vi "4.0.0_Self Test.vi"(7 "Data in":T1, 8 "error in (no error)":errorcluster, 9 "AllControls In":T2, 10 "?":T3, 11 "Message Queue out":T4) -> (0 "error out":errorcluster, 1 "Flow":string, 2 "Data":T3, 3 "Message Queue Out":T4, 5 "Data out":T1)   [LabVIEW 2017]
uses:
  Depends/AMC/subVIs/TypeDefs/amc_Message Queue.ctl
  Depends/AMC/subVIs/TypeDefs/amc_Message.ctl
  Depends/Tools/Keyed Array/Tools_KeyedArray KeyedArray.ctl
  Ctrls/Data.ctl
  Ctrls/AllControls.ctl
  Ctrls/CSV_Data.ctl
  DIPC 692 Daemon API/typdef/destination.ctl
  DIPC 692 Daemon API/typdef/device_mode.ctl
  Ctrls/PathChoose.ctl
  DIPC 692 Daemon API/typdef/read_nvm_section.ctl
  DIPC 692 Daemon API/typdef/get_parameter.ctl
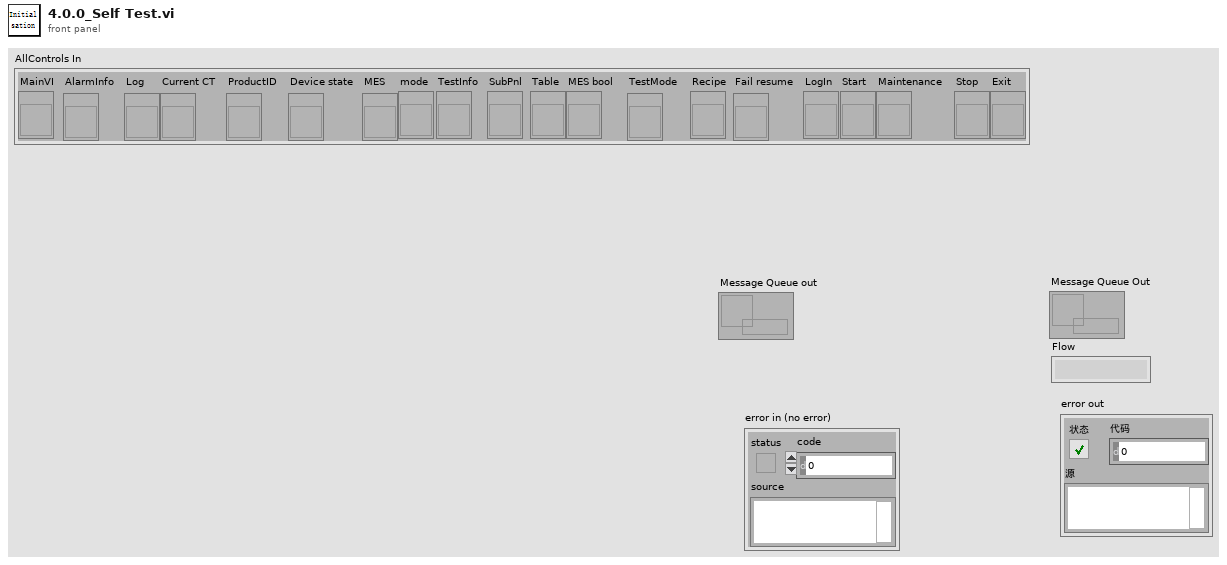
[diagram p1: front panel]
types:
  T1 = typedef "CSV_Data.ctl" = cluster{"Initialisation":cluster{"LMT - Connect UUT (con COM)":string, "LMT - Software Version (rrel)":string, "LMT - Write SKU file (wskuc)":string, "LMT - SKU file name":string, "Connect UUT DDM":string, "Read DDM EOL Timestamp - Mode":string, "Read DDM EOL Timestamp - Timestamp":string, "Read DDM EOL Timestamp - Rig ID":string, "Read DDM EOL Timestamp - Passmark ID":string, "Read DDM EOL Timestamp - Passmark Rev":string, "Software Version before flashing":string, "Read Hardware Serial":string, "UUT DDM SN":string, "Compare DDM SN with MES SN":string, "Backup PCBA Calibration EEPROM Response - CAL":string, "Flash Firmware Version":string, "Check SW Version":string, "Read DDM SW Version after flashing":string, "Set SKU Config":string, "Ready Status":string, "Set Device Mode to EOL":string, "DDM Parameter - Voltage":string, "DDM Parameter - Current":string, "DDM Parameter - Power":string, "DDM Parameter - Speed":string, "DDM Parameter - Pressure":string, "Tester Parameter - Voltage":string, "Tester Parameter - Current":string, "Tester Parameter - Power":string, "Tester Parameter - Ambient Pressure":string, "Tester Parameter - Ambient Temperature":string, "Calculated Parameter - DDM Pressure Corrected":string, "Calculated Parameter - DDM Real Power":string, "Calculated Parameter - Delta V":string}, "BEMF_Calibration":cluster{"Calibration Result - eol_cold_bemf_temp":string, "DDM Ambient Temp":string, "Restriction Plate Diameter":string, "Calibration Result - eol_bemf_mp_cold_coef_a":string, "Calibration Result - eol_bemf_mp_cold_coef_b":string, "Calibration Result - eol_bemf_mp_cold_coef_c":string, "Calibration Result - eol_bemf_lsi_cold_ref_coeffs":string, "Get - Calibration Result - eol_bemf_lsi_speed":string, "Get - Calibration Result - eol_bemf_lsi_integral_0":string, "Calibration Result - eol_bemf_lsi_integral_1":string, "Get - Calibration Result - eol_bemf_lsi_integral_2":string, "Get - Calibration Result - eol_cold_bemf":string, "Get - Calibration Result - eol_cold_bemf_fisf":string, "Finalise Calibration":string, "Compare -Calibration Result - eol_cold_bemf":string, "Compare -Calibration Result - eol_cold_bemf_fisf":string}, "ECO":cluster{"Reset Power Tune":string, "Reset BEMF FISF Calibration":string, "Restriction Plate Diameter":string, "ECO - Stabilisation Time":string, "ECO - DDM Parameter - Voltage":string, "ECO - DDM Parameter - Current":string, "ECO - DDM Parameter - Power":string, "ECO - DDM Parameter - Measured Power":string, "ECO - DDM Parameter - Speed":string, "ECO - DDM Parameter - Pressure":string, "ECO - Tester Parameter - Voltage":string, "ECO - Tester Parameter - Current":string, "ECO - Tester Parameter - Power":string, "ECO - Tester Parameter - Ambient Pressure":string, "ECO - Tester Parameter - Ambient Temperature":string, "ECO - Tester Parameter - Ambient Humidity":string, "ECO - Calculated Parameter - DDM Pressure Corrected":string, "ECO - Calculated Parameter - DDM Real Power":string, "ECO - Calculated Parameter - Delta V":string, "ECO - Calculated Parameter - Flowrate":string, "ECO - Calculated Parameter - Airwatt":string, "ECO - Formula":string, "PT ECO - Power Tune Mode Status":string}, "BOOST":cluster{"Restriction Plate Diameter":string, "BOOST - Stabilisation Time":string, "BOOST - DDM Parameter - Voltage":string, "BOOST - DDM Parameter - Current":string, "BOOST - DDM Parameter - Power":string, "BOOST - DDM Parameter - Measured Power":string, "BOOST - DDM Parameter - Speed":string, "BOOST - DDM Parameter - Pressure":string, "BOOST - Tester Parameter - Voltage":string, "BOOST - Tester Parameter - Current":string, "BOOST - Tester Parameter - Power":string, "BOOST - Tester Parameter - Ambient Pressure":string, "BOOST - Tester Parameter - Ambient Temperature":string, "BOOST - Tester Parameter - Ambient Humidity":string, "BOOST - Calculated Parameter - DDM Pressure Corrected":string, "BOOST - Calculated Parameter - DDM Real Power":string, "BOOST - Calculated Parameter - Delta V":string, "BOOST - Calculated Parameter - Flowrate":string, "BOOST - Calculated Parameter - Airwatt":string, "BOOST - Get AM Presence":string, "Air Muscle Turn Off Status":string, "BOOST - Air Muscle Calculated Parameter - Airwatt B":string, "BOOST - Air Muscle Calculate Airwatt Delta":string, "PT BOOST - Power Tune Mode Status":string, "Finalise Calibration":string, "ECO - Get AW Calibration value":string, "BOOST - Get AW Calibration value":string}, "MAX":cluster{"Restriction Plate Diameter":string, "MAX - Stabilisation Time":string, "Get Average Delta Tmag (LSIdelta_FISFdelta_LSItmag_FISFtmag_IIRtmag)":string, "Get Average Delta Tmag FISF":string, "MAX - DDM Parameter - Voltage":string, "MAX - DDM Parameter - Current":string, "MAX - DDM Parameter - Power":string, "MAX - DDM Parameter - Measured Power":string, "MAX - DDM Parameter - Speed":string, "MAX - DDM Parameter - Pressure":string, "MAX - Tester Parameter - Voltage":string, "MAX - Tester Parameter - Current":string, "MAX - Tester Parameter - Power":string, "MAX - Tester Parameter - Ambient Pressure":string, "MAX - Tester Parameter - Ambient Temperature":string, "MAX - Tester Parameter - Ambient Humidity":string, "MAX - Calculated Parameter - DDM Pressure Corrected":string, "MAX - Calculated Parameter - DDM Real Power":string, "MAX - Calculated Parameter - Delta V":string, "MAX - Calculated Parameter - Flowrate":string, "MAX - Calculated Parameter - Airwatt":string, "MAX_FISF_Check_Average_Delta_Tmag":string, "MAX - FISF - BEMF Finetune Result":string, "MAX tune - Delta P1":string, "MAX tune - Calculated Parameter - Airwatt":string, "Calculate Delta Airwatts - MAX finetune - Delta P2":string, "MAX finetune - DDM Parameter - Voltage":string, "MAX finetune - DDM Parameter - Current":string, "MAX finetune - DDM Parameter - Power":string, "MAX finetune - DDM Parameter - Measured Power":string, "MAX finetune - DDM Parameter - Speed":string, "MAX finetune - DDM Parameter - Pressure":string, "MAX finetune - Tester Parameter - Voltage":string, "MAX finetune - Tester Parameter - Current":string, "MAX finetune - Tester Parameter - Power":string, "MAX finetune - Tester Parameter - Ambient Pressure":string, "MAX finetune - Tester Parameter - Ambient Temperature":string, "MAX finetune - Tester Parameter - Ambient Humidity":string, "MAX finetune - Calculated Parameter - DDM Pressure Corrected":string, "MAX finetune - Calculated Parameter - DDM Real Power":string, "MAX finetune - Calculated Parameter - Delta V":string, "MAX finetune - Calculated Parameter - Flowrate":string, "MAX finetune - Calculated Parameter - Airwatt":string, "Check Derate Result":string, "Delta Tmag FISF":string, "Get Hot BEMF Result":string, "Calculate delta Pressure":string, "Finalise Calibration":string, "Calculate & Check Delta BEMF":string, "Delta P Airwatts Value":string}, "LL":cluster{"DDM Ambient Temp":string, "Restriction Plate Diameter":string, "LL - DDM Parameter - Voltage":string, "LL - DDM Parameter - Current":string, "LL - DDM Parameter - Power":string, "LL - DDM Parameter - Measured Power":string, "LL - DDM Parameter - Speed":string, "LL - DDM Parameter - Pressure":string, "LL - Tester Parameter - Voltage":string, "LL - Tester Parameter - Current":string, "LL - Tester Parameter - Power":string, "LL - DDM Real Power":string, "LL - Calibrate Task Detect LL":string}, "HL":cluster{"HL - DDM Parameter - Voltage":string, "HL - DDM Parameter - Current":string, "HL - DDM Parameter - Power":string, "HL - DDM Parameter - Measured Power":string, "HL - DDM Parameter - Speed":string, "HL - DDM Parameter - Pressure":string, "HL - Tester Parameter - Voltage":string, "HL - Tester Parameter - Current":string, "HL - Tester Parameter - Power":string, "HL - DDM Real Power":string, "HL - Calibrate Task Detect HL":string}, "LH":cluster{"Restriction Plate Diameter":string, "LH - DDM Parameter - Voltage":string, "LH - DDM Parameter - Current":string, "LH - DDM Parameter - Power":string, "LH - DDM Parameter - Measured Power":string, "LH - DDM Parameter - Speed":string, "LH - DDM Parameter - Pressure":string, "LH - Tester Parameter - Voltage":string, "LH - Tester Parameter - Current":string, "LH - Tester Parameter - Power":string, "LH - DDM Real Power":string, "LH - Calibrate Task Detect LH":string}, "HH":cluster{"HH - DDM Parameter - Voltage":string, "HH - DDM Parameter - Current":string, "HH - DDM Parameter - Power":string, "HH - DDM Parameter - Measured Power":string, "HH - DDM Parameter - Speed":string, "HH - DDM Parameter - Pressure":string, "HH - Tester Parameter - Voltage":string, "HH - Tester Parameter - Current":string, "HH - Tester Parameter - Power":string, "HH - DDM Real Power":string, "HH - Calibrate Task Detect HH":string}, "Inlet Blockage Calibration":cluster{"Inlet Blockage Calibration - DDM Parameter - Voltage":string, "Inlet Blockage Calibration - DDM Parameter - Current":string, "Inlet Blockage Calibration - DDM Parameter - Power":string, "Inlet Blockage Calibration - DDM Parameter - Measured Power":string, "Inlet Blockage Calibration - DDM Parameter - Speed":string, "Inlet Blockage Calibration - DDM Parameter - Pressure":string, "Inlet Blockage Calibration - Tester Parameter - Voltage":string, "Inlet Blockage Calibration - Tester Parameter - Current":string, "Inlet Blockage Calibration - Tester Parameter - Power":string, "Inlet Blockage Calibration - DDM Real Power":string, "Calibration Inlet Blockage_E":string, "Finalise Calibration":string, "Get Task Detect LL":string, "Get Task Detect HL":string, "Get Task Detect LH":string, "Get Task Detect HH":string, "Calibration Inlet Blockage":string, "Calibration eol cold bemf temp":string}, "GOOD":cluster{"GOOD UNIT - Clear EEPROM Error Log":string, "GOOD UNIT - Write Product Timestamp - Mode":string, "GOOD UNIT - Write Product Timestamp - Timestamp":string, "GOOD UNIT - Write Product Timestamp - Rig ID":string, "GOOD UNIT - Write Product Timestamp - Passmark ID":string, "GOOD UNIT - Write Product Timestamp - Passmark Rev":string, "GOOD UNIT - Set Device Mode to PROD":string, "GOOD UNIT - Backup PCBA Calibration EEPROM Response":string, "GOOD UNIT - Check Security Bit":string, "GOOD UNIT - Set Calibration Lock":string, "GOOD UNIT - Get_Calibration_Lock":string, "GOOD UNIT - Disconnect UUT":string}, "NG":cluster{"NG UNIT - Read NVM Error":string, "NG UNIT - Set Device Mode to FCT":string, "NG UNIT - Backup PCBA Calibration EEPROM Response - CAL":string, "NG UNIT - Backup PCBA Calibration EEPROM Response - ERROR":string, "NG UNIT - Backup PCBA Calibration EEPROM Response - USAGE":string, "NG UNIT - Disconnect UUT":string}, "SN":string, "Table":string[][], "Count":cluster{"Total":i32, "OK":i32, "NG":i32, "Yield":dbl}, "Start Time":timestamp, "daemon reference":refnum<k5>, "CT":dbl, "Config":string[][], "OK/NG":bool, "Station ID":string, "MES DDM SN":string, "MES PCBA SN":string, "Retest":string, "Lux":string, "Initialisation_Status":cluster{"LMT - Connect UUT (con COM)":string, "LMT - Software Version (rrel)":string, "LMT - Write SKU file (wskuc)":string, "LMT - SKU file name":string, "Connect UUT DDM":string, "Read DDM EOL Timestamp - Mode":string, "Read DDM EOL Timestamp - Timestamp":string, "Read DDM EOL Timestamp - Rig ID":string, "Read DDM EOL Timestamp - Passmark ID":string, "Read DDM EOL Timestamp - Passmark Rev":string, "Software Version before flashing":string, "Read Hardware Serial":string, "UUT DDM SN":string, "Compare DDM SN with MES SN":string, "Backup PCBA Calibration EEPROM Response - CAL":string, "Flash Firmware Version":string, "Check SW Version":string, "Read DDM SW Version after flashing":string, "Set SKU Config":string, "Ready Status":string, "Set Device Mode to EOL":string, "DDM Parameter - Voltage":string, "DDM Parameter - Current":string, "DDM Parameter - Power":string, "DDM Parameter - Speed":string, "DDM Parameter - Pressure":string, "Tester Parameter - Voltage":string, "Tester Parameter - Current":string, "Tester Parameter - Power":string, "Tester Parameter - Ambient Pressure":string, "Tester Parameter - Ambient Temperature":string, "Calculated Parameter - DDM Pressure Corrected":string, "Calculated Parameter - DDM Real Power":string, "Calculated Parameter - Delta V":string}, "BEMF_Calibration_Status":cluster{"Calibration Result - eol_cold_bemf_temp":string, "DDM Ambient Temp":string, "Restriction Plate Diameter":string, "Calibration Result - eol_bemf_mp_cold_coef_a":string, "Calibration Result - eol_bemf_mp_cold_coef_b":string, "Calibration Result - eol_bemf_mp_cold_coef_c":string, "Calibration Result - eol_bemf_lsi_cold_ref_coeffs":string, "Get - Calibration Result - eol_bemf_lsi_speed":string, "Get - Calibration Result - eol_bemf_lsi_integral_0":string, "Calibration Result - eol_bemf_lsi_integral_1":string, "Get - Calibration Result - eol_bemf_lsi_integral_2":string, "Get - Calibration Result - eol_cold_bemf":string, "Get - Calibration Result - eol_cold_bemf_fisf":string, "Finalise Calibration":string, "Compare -Calibration Result - eol_cold_bemf":string, "Compare -Calibration Result - eol_cold_bemf_fisf":string}, "ECO_Status":cluster{"Reset Power Tune":string, "Reset BEMF FISF Calibration":string, "Restriction Plate Diameter":string, "ECO - Stabilisation Time":string, "ECO - DDM Parameter - Voltage":string, "ECO - DDM Parameter - Current":string, "ECO - DDM Parameter - Power":string, "ECO - DDM Parameter - Measured Power":string, "ECO - DDM Parameter - Speed":string, "ECO - DDM Parameter - Pressure":string, "ECO - Tester Parameter - Voltage":string, "ECO - Tester Parameter - Current":string, "ECO - Tester Parameter - Power":string, "ECO - Tester Parameter - Ambient Pressure":string, "ECO - Tester Parameter - Ambient Temperature":string, "ECO - Tester Parameter - Ambient Humidity":string, "ECO - Calculated Parameter - DDM Pressure Corrected":string, "ECO - Calculated Parameter - DDM Real Power":string, "ECO - Calculated Parameter - Delta V":string, "ECO - Calculated Parameter - Flowrate":string, "ECO - Calculated Parameter - Airwatt":string, "ECO - Formula":string, "PT ECO - Power Tune Mode Status":string}, "BOOST_Status":cluster{"Restriction Plate Diameter":string, "BOOST - Stabilisation Time":string, "BOOST - DDM Parameter - Voltage":string, "BOOST - DDM Parameter - Current":string, "BOOST - DDM Parameter - Power":string, "BOOST - DDM Parameter - Measured Power":string, "BOOST - DDM Parameter - Speed":string, "BOOST - DDM Parameter - Pressure":string, "BOOST - Tester Parameter - Voltage":string, "BOOST - Tester Parameter - Current":string, "BOOST - Tester Parameter - Power":string, "BOOST - Tester Parameter - Ambient Pressure":string, "BOOST - Tester Parameter - Ambient Temperature":string, "BOOST - Tester Parameter - Ambient Humidity":string, "BOOST - Calculated Parameter - DDM Pressure Corrected":string, "BOOST - Calculated Parameter - DDM Real Power":string, "BOOST - Calculated Parameter - Delta V":string, "BOOST - Calculated Parameter - Flowrate":string, "BOOST - Calculated Parameter - Airwatt":string, "BOOST - Get AM Presence":string, "Air Muscle Turn Off Status":string, "BOOST - Air Muscle Calculated Parameter - Airwatt B":string, "BOOST - Air Muscle Calculate Airwatt Delta":string, "PT BOOST - Power Tune Mode Status":string, "Finalise Calibration":string, "ECO - Get AW Calibration value":string, "BOOST - Get AW Calibration value":string}, "MAX_Status":cluster{"Restriction Plate Diameter":string, "MAX - Stabilisation Time":string, "Get Average Delta Tmag (LSIdelta_FISFdelta_LSItmag_FISFtmag_IIRtmag)":string, "Get Average Delta Tmag FISF":string, "MAX - DDM Parameter - Voltage":string, "MAX - DDM Parameter - Current":string, "MAX - DDM Parameter - Power":string, "MAX - DDM Parameter - Measured Power":string, "MAX - DDM Parameter - Speed":string, "MAX - DDM Parameter - Pressure":string, "MAX - Tester Parameter - Voltage":string, "MAX - Tester Parameter - Current":string, "MAX - Tester Parameter - Power":string, "MAX - Tester Parameter - Ambient Pressure":string, "MAX - Tester Parameter - Ambient Temperature":string, "MAX - Tester Parameter - Ambient Humidity":string, "MAX - Calculated Parameter - DDM Pressure Corrected":string, "MAX - Calculated Parameter - DDM Real Power":string, "MAX - Calculated Parameter - Delta V":string, "MAX - Calculated Parameter - Flowrate":string, "MAX - Calculated Parameter - Airwatt":string, "MAX_FISF_Check_Average_Delta_Tmag":string, "MAX - FISF - BEMF Finetune Result":string, "MAX tune - Delta P1":string, "MAX tune - Calculated Parameter - Airwatt":string, "Calculate Delta Airwatts - MAX finetune - Delta P2":string, "MAX finetune - DDM Parameter - Voltage":string, "MAX finetune - DDM Parameter - Current":string, "MAX finetune - DDM Parameter - Power":string, "MAX finetune - DDM Parameter - Measured Power":string, "MAX finetune - DDM Parameter - Speed":string, "MAX finetune - DDM Parameter - Pressure":string, "MAX finetune - Tester Parameter - Voltage":string, "MAX finetune - Tester Parameter - Current":string, "MAX finetune - Tester Parameter - Power":string, "MAX finetune - Tester Parameter - Ambient Pressure":string, "MAX finetune - Tester Parameter - Ambient Temperature":string, "MAX finetune - Tester Parameter - Ambient Humidity":string, "MAX finetune - Calculated Parameter - DDM Pressure Corrected":string, "MAX finetune - Calculated Parameter - DDM Real Power":string, "MAX finetune - Calculated Parameter - Delta V":string, "MAX finetune - Calculated Parameter - Flowrate":string, "MAX finetune - Calculated Parameter - Airwatt":string, "Check Derate Result":string, "Delta Tmag FISF":string, "Get Hot BEMF Result":string, "Calculate delta Pressure":string, "Finalise Calibration":string, "Calculate & Check Delta BEMF":string, "Delta P Airwatts Value":string}, "LL_Status":cluster{"DDM Ambient Temp":string, "Restriction Plate Diameter":string, "LL - DDM Parameter - Voltage":string, "LL - DDM Parameter - Current":string, "LL - DDM Parameter - Power":string, "LL - DDM Parameter - Measured Power":string, "LL - DDM Parameter - Speed":string, "LL - DDM Parameter - Pressure":string, "LL - Tester Parameter - Voltage":string, "LL - Tester Parameter - Current":string, "LL - Tester Parameter - Power":string, "LL - DDM Real Power":string, "LL - Calibrate Task Detect LL":string}, "HL_Status":cluster{"HL - DDM Parameter - Voltage":string, "HL - DDM Parameter - Current":string, "HL - DDM Parameter - Power":string, "HL - DDM Parameter - Measured Power":string, "HL - DDM Parameter - Speed":string, "HL - DDM Parameter - Pressure":string, "HL - Tester Parameter - Voltage":string, "HL - Tester Parameter - Current":string, "HL - Tester Parameter - Power":string, "HL - DDM Real Power":string, "HL - Calibrate Task Detect HL":string}, "LH_Status":cluster{"Restriction Plate Diameter":string, "LH - DDM Parameter - Voltage":string, "LH - DDM Parameter - Current":string, "LH - DDM Parameter - Power":string, "LH - DDM Parameter - Measured Power":string, "LH - DDM Parameter - Speed":string, "LH - DDM Parameter - Pressure":string, "LH - Tester Parameter - Voltage":string, "LH - Tester Parameter - Current":string, "LH - Tester Parameter - Power":string, "LH - DDM Real Power":string, "LH - Calibrate Task Detect LH":string}, "HH_Status":cluster{"HH - DDM Parameter - Voltage":string, "HH - DDM Parameter - Current":string, "HH - DDM Parameter - Power":string, "HH - DDM Parameter - Measured Power":string, "HH - DDM Parameter - Speed":string, "HH - DDM Parameter - Pressure":string, "HH - Tester Parameter - Voltage":string, "HH - Tester Parameter - Current":string, "HH - Tester Parameter - Power":string, "HH - DDM Real Power":string, "HH - Calibrate Task Detect HH":string}, "Inlet Blockage Calibration_Status":cluster{"Inlet Blockage Calibration - DDM Parameter - Voltage":string, "Inlet Blockage Calibration - DDM Parameter - Current":string, "Inlet Blockage Calibration - DDM Parameter - Power":string, "Inlet Blockage Calibration - DDM Parameter - Measured Power":string, "Inlet Blockage Calibration - DDM Parameter - Speed":string, "Inlet Blockage Calibration - DDM Parameter - Pressure":string, "Inlet Blockage Calibration - Tester Parameter - Voltage":string, "Inlet Blockage Calibration - Tester Parameter - Current":string, "Inlet Blockage Calibration - Tester Parameter - Power":string, "Inlet Blockage Calibration - DDM Real Power":string, "Calibration Inlet Blockage_E":string, "Finalise Calibration":string, "Get Task Detect LL":string, "Get Task Detect HL":string, "Get Task Detect LH":string, "Get Task Detect HH":string, "Calibration Inlet Blockage":string, "Calibration eol cold bemf temp":string}, "GOOD_Status":cluster{"GOOD UNIT - Clear EEPROM Error Log":string, "GOOD UNIT - Write Product Timestamp - Mode":string, "GOOD UNIT - Write Product Timestamp - Timestamp":string, "GOOD UNIT - Write Product Timestamp - Rig ID":string, "GOOD UNIT - Write Product Timestamp - Passmark ID":string, "GOOD UNIT - Write Product Timestamp - Passmark Rev":string, "GOOD UNIT - Set Device Mode to PROD":string, "GOOD UNIT - Backup PCBA Calibration EEPROM Response":string, "GOOD UNIT - Check Security Bit":string, "GOOD UNIT - Set Calibration Lock":string, "GOOD UNIT - Get_Calibration_Lock":string, "GOOD UNIT - Disconnect UUT":string}, "NG_Status":cluster{"NG UNIT - Read NVM Error":string, "NG UNIT - Set Device Mode to FCT":string, "NG UNIT - Backup PCBA Calibration EEPROM Response - CAL":string, "NG UNIT - Backup PCBA Calibration EEPROM Response - ERROR":string, "NG UNIT - Backup PCBA Calibration EEPROM Response - USAGE":string, "NG UNIT - Disconnect UUT":string}, "SKU":string, "Plate_Diameter":string, "Alarm":string}
  T2 = typedef "AllControls.ctl" = cluster{"MainVI":refnum<vi>, "AlarmInfo":refnum<vi>, "Log":refnum<vi>, "Current CT":refnum<vi>, "ProductID":refnum<vi>, "Device state":refnum<vi>, "MES":refnum<vi>, "mode":refnum<vi>, "TestInfo":refnum<vi>, "SubPnl":refnum<vi>, "Table":refnum<vi>, "MES bool":refnum<vi>, "TestMode":refnum<vi>, "Recipe":refnum<vi>, "Fail resume":refnum<vi>, "LogIn":refnum<vi>, "Start":refnum<vi>, "Maintenance":refnum<vi>, "Stop":refnum<vi>, "Exit":refnum<vi>}
  T3 = typedef "Data.ctl" = cluster{"Initialisation":cluster{"DDM_Parameter":dbl[], "DDM_Parameter_status":bool[], "Get_Tester_Parameter":dbl[], "Get_Tester_Parameter_status":bool[], "Cal_Tester_Parameter":dbl[], "Cal_Tester_Parameter_status":bool[], "sw_version_before_status":bool, "sw_version_after_status":bool, "Set_SKU_Config_With_LMT_status":bool, "FCT_timestamp_status":bool, "LMT_Connect_to_UUT_status":bool}, "BEMF_Calibration":cluster{"Read_ambient_temperature":dbl, "Calibration_Vaule":dbl[], "Calibration_Vaule _B":dbl[], "Calibration_Vaule_status":bool[], "Calibration_Vaule_B_status":bool[]}, "ECO":cluster{"DDM_Parameter":dbl[], "DDM_Parameter_status":bool[], "Get_Tester_Parameter":dbl[], "Get_Tester_Parameter_status":bool[], "Cal_Tester_Parameter":dbl[], "Cal_Tester_Parameter_status":bool[], "DDM_Parameter_after_power_tune":dbl[], "Get_Tester_Parameter_after_power_tune":dbl[], "Cal_Tester_Parameter_after_power_tune":dbl[], "Cal_Tester_Parameter_after_power_tune_status":bool[], "Delta_P":dbl}, "BOOST":cluster{"DDM_Parameter":dbl[], "DDM_Parameter_status":bool[], "Get_Tester_Parameter":dbl[], "Get_Tester_Parameter_status":bool[], "Cal_Tester_Parameter":dbl[], "Cal_Tester_Parameter_status":bool[], "DDM_Parameter_after_power_tune":dbl[], "Get_Tester_Parameter_after_power_tune":dbl[], "Cal_Tester_Parameter_after_power_tune":dbl[], "Cal_Tester_Parameter_after_power_tune_status":bool[], "airwatts_am_off":dbl, "AW_Delta_(AM_on_and_off)":dbl, "AW_Delta_(AM_on_and_off)_Status":bool, "Delta_P":dbl}, "MAX":cluster{"Average_Tmag_Data":cluster{"LSI Delta in degC":dbl, "FISF Delta in degc":dbl, "LSI Tmag in degC":dbl, "Fisf Tmag in degC":dbl, "IIR Tmag in degC":dbl}, "DDM_Parameter":dbl[], "DDM_Parameter_status":bool[], "Get_Tester_Parameter":dbl[], "Get_Tester_Parameter_status":bool[], "Cal_Tester_Parameter":dbl[], "BEMF_Finetune":cluster{"eol_bemf_mp_cold_coef_c":dbl, "eol_cold_bemf_fisf_offset":dbl}, "AW_Tune":cluster{"delta_P1":dbl, "delta_P_Setting":dbl}, "DDM_Parameter_after_Airwatts_Tune":dbl[], "Get_Tester_Parameter_after_Airwatts_Tune":dbl[], "Cal_Tester_Parameter_after_Airwatts_Tune":dbl[], "DDM_Parameter_after_Airwatts_Finetune":dbl[], "Get_Tester_Parameter_after_Airwatts_Finetune":dbl[], "Cal_Tester_Parameter_after_Airwatts_Finetune":dbl[], "AW_Finetune":cluster{"delta_P2":dbl, "delta_P_Setting":dbl}, "Delta_Tmag_after_tune":cluster{"LSI Delta in degC":dbl, "FISF Delta in degc":dbl, "LSI Tmag in degC":dbl, "Fisf Tmag in degC":dbl, "IIR Tmag in degC":dbl}, "Hot Bemf in mV":dbl, "DDM_Pressure":dbl, "Delta_Pressure":dbl, " Cold Bemf in mV":dbl, " delta Bemf":dbl, " delta p":dbl, "Delta_Pressure_status":bool, " delta Bemf_status":bool, "LSI Delta in degC_status":bool, "FISF Delta in degc_status":bool, "Max_check_derate_status_status":bool, "Average_All_data":dbl[][], "Average_Tmag_Data_status":bool[], "Average_Tmag_Data_after_tune_status":bool[], "Cal_Tester_Parameter_status":bool[], "Cal_Tester_Parameter_status_after_Airwatts_Tune":bool[], "Cal_Tester_Parameter_status_after_Airwatts_FineTune":bool[]}, "Task_Detect_Calib":cluster{"LL":cluster{"DDM_Parameter":dbl[], "DDM_Parameter_status":bool[], "Get_Tester_Parameter":dbl[], "Get_Tester_Parameter_status":bool[], "Set_task_detect_A":dbl, "Set_task_detect_A_Status":bool}, "HL":cluster{"DDM_Parameter":dbl[], "DDM_Parameter_status":bool[], "Get_Tester_Parameter":dbl[], "Get_Tester_Parameter_status":bool[], "Set_task_detect_B":dbl, "Set_task_detect_B_Status":bool}, "LH":cluster{"DDM_Parameter":dbl[], "DDM_Parameter_status":bool[], "Get_Tester_Parameter":dbl[], "Get_Tester_Parameter_status":bool[], "Set_task_detect_C":dbl, "Set_task_detect_C_Status":bool}, "HH":cluster{"DDM_Parameter":dbl[], "DDM_Parameter_status":bool[], "Get_Tester_Parameter":dbl[], "Get_Tester_Parameter_status":bool[], "Set_task_detect_D":dbl, "Read_and_check_calibration_Status":bool[], "Set_task_detect_D_Status":bool}, "Get_eol_inlet_blockage_E":dbl, "Calib_vaule":cluster{"Get_task_detect_LL":dbl, "Get_task_detect_HL":dbl, "Get_task_detect_LH":dbl, "Get_task_detect_HH":dbl, "eol_inlet_blockage":dbl, "eol_code_bemf_temp":dbl}, "calibrated temp":dbl, "Inlet_Blockage_Calibration":cluster{"DDM_Parameter":dbl[], "DDM_Parameter_status":bool[], "Get_Tester_Parameter":dbl[], "Get_Tester_Parameter_status":bool[]}, "Get_eol_inlet_blockage_E_Status":bool}, "good":cluster{"Write_Product_TS":cluster{"TIMESTAMP":i64, "RIG_ID":i64, "PASSMARK_ID":i64, "PASSMARK_REV":i64}, "Read_Product_TS":cluster{"TIMESTAMP":i64, "RIG_ID":i64, "PASSMARK_ID":i64, "PASSMARK_REV":i64}, "Good_Check_Secuity_Bit_Stauts":bool}}
  T4 = typedef "amc_Message Queue.ctl" = refnum<queue>
  T5 = cluster{"Brush_ADC.bat":string, "Get Release Version.bat":string, "Getting Software  Version.bat":string, "Pump_ADC.bat":string, "Starting  Pump Motor.bat":string, "Starting  Test Mode.bat":string, "Starting Brush Motor 1.bat":string, "Starting Brush Motor 2.bat":string, "Starting Brush Motor 3.bat":string, "Starting LED Test.bat":string, "Stopping  Brush Motor.bat":string, "Stopping  Pump Motor.bat":string, "Stopping  Test Mode.bat":string, "1":string, "2":string, "3":string, "4":string, "5":string, "6":string, "7":string, "8":string, "9":string, "10":string}
  T6 = typedef "destination.ctl" = string
  T7 = typedef "PathChoose.ctl" = enum16{"OperatorLog", "AutoRunLog", "AlmLog", "TestData", "AllTestData", "backup_nvm", "backup_before_flashing"}
  T8 = enum16{"open", "replace", "create", "open or create", "replace or create", "replace or create with confirmation"}
  T9 = typedef "read_nvm_section.ctl" = enum16{"CAL", "ERROR", "USAGE"}
  T10 = typedef "get_parameter.ctl" = string
  T11 = typedef "HD Config.ctl" = cluster{" PC":cluster{"PC Address":u8[], "PC Port":i32}, "FCO":cluster{"COM":refnum<visa-resource-name>, "Baudrate":u32}, "DC Power ":cluster{"COM":refnum<visa-resource-name>, "Baudrate":u32}, "PW3336":cluster{"COM":refnum<visa-resource-name>, "Baudrate":u32}, "Lefoo":cluster{"COM":refnum<visa-resource-name>, "Baudrate":u32}, "Tempt&Hum":cluster{"COM":refnum<visa-resource-name>, "Baudrate":u32}, "DIPC":cluster{"COM":refnum<visa-resource-name>}, "Daemon":cluster{"IP Address":string, "Port":u16, "Retry":u16}, "URAT":cluster{"COM":refnum<visa-resource-name>, "Baudrate":u32}, "Fail_resume_mode":bool, "GRR":bool}
  T12 = typedef "device_mode.ctl" = enum16{"FCT", "EOL", "PROD"}
  T13 = cluster{"TIMESTAMP":i64, "RIG_ID":i64, "PASSMARK_ID":i64, "PASSMARK_REV":i64}
  T14 = cluster{"TIMESTAMP":string, "RIG_ID":string, "PASSMARK_ID":string, "PASSMARK_REV":string}
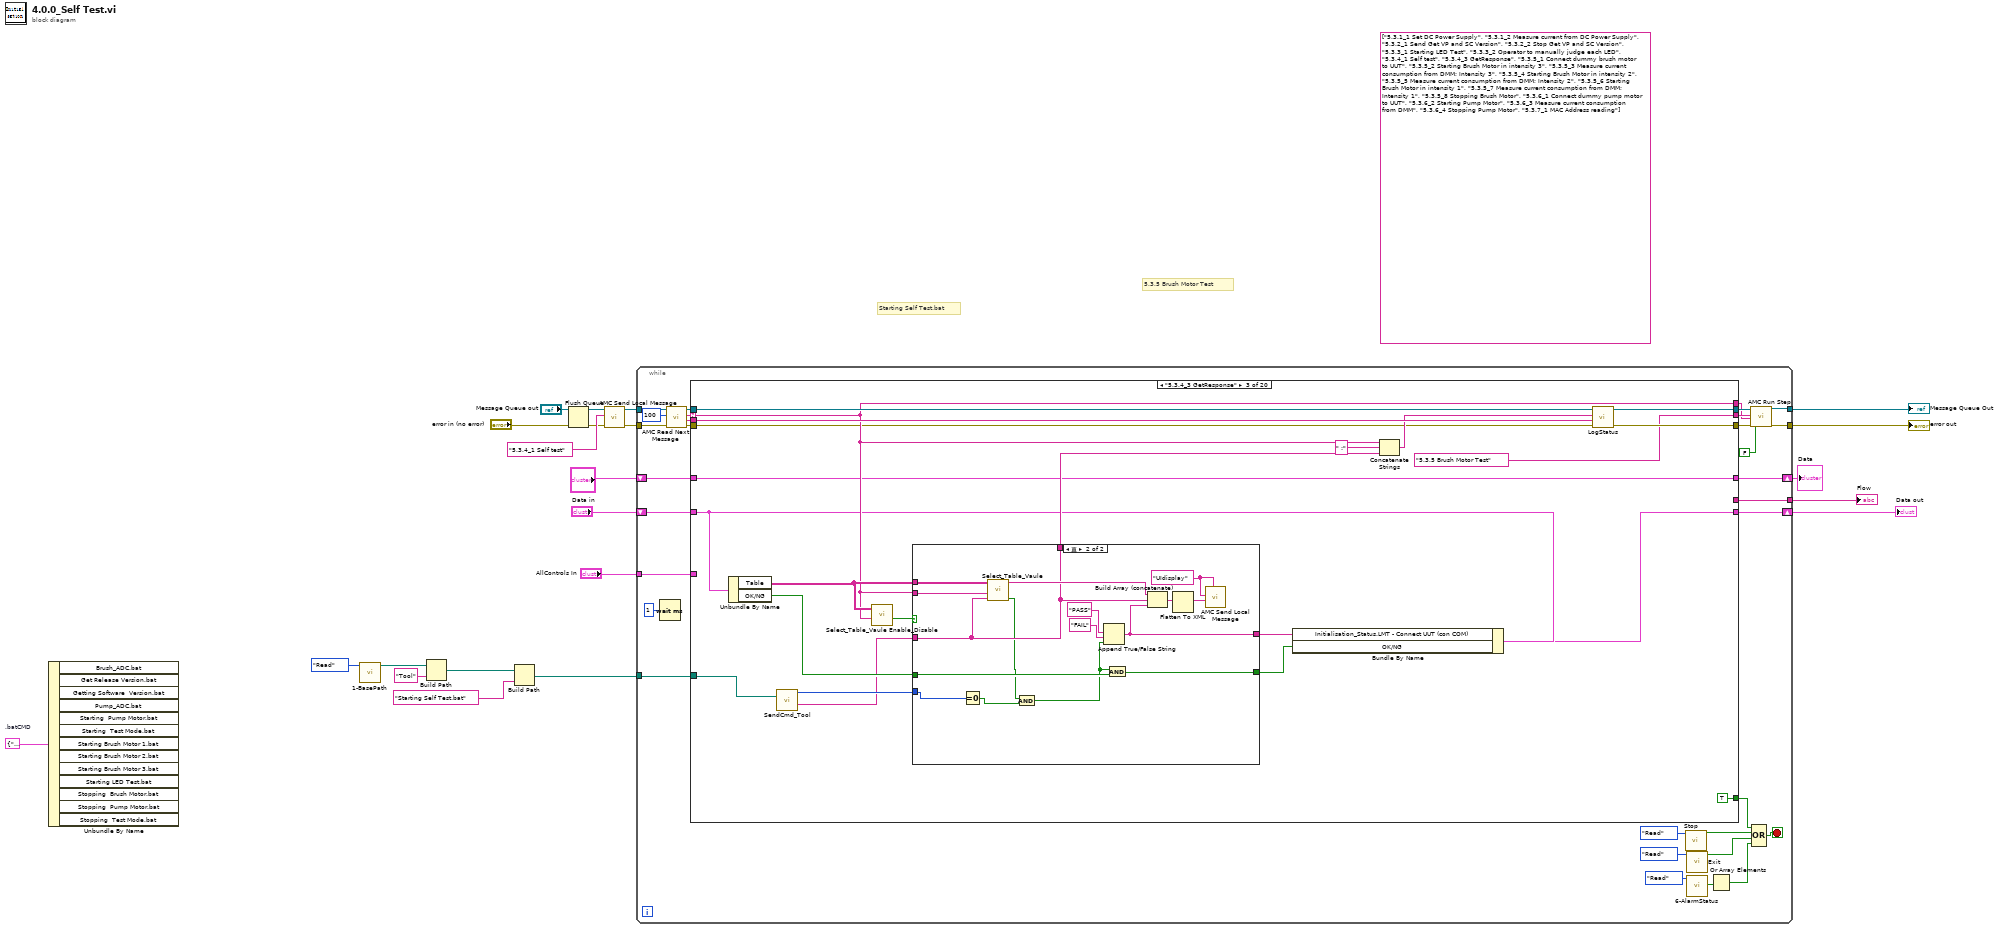
[diagram p0: block diagram]
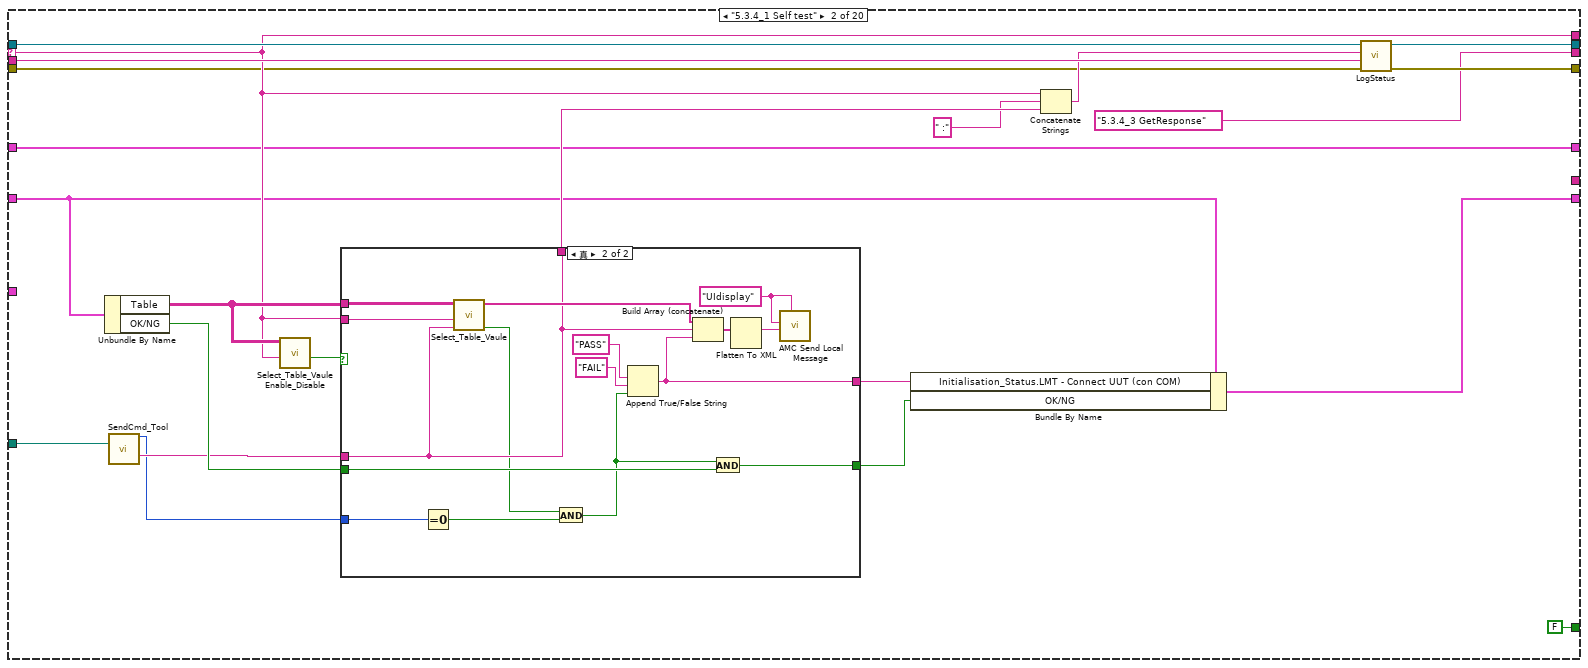
[diagram p3: hidden frame]
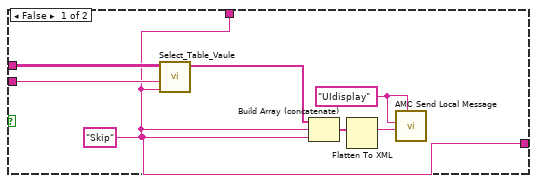
[diagram p4: hidden frame]
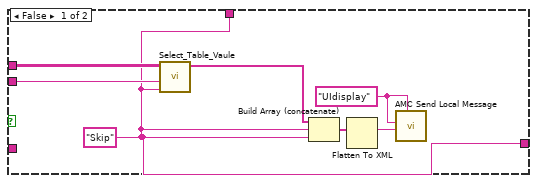
[diagram p5: hidden frame]
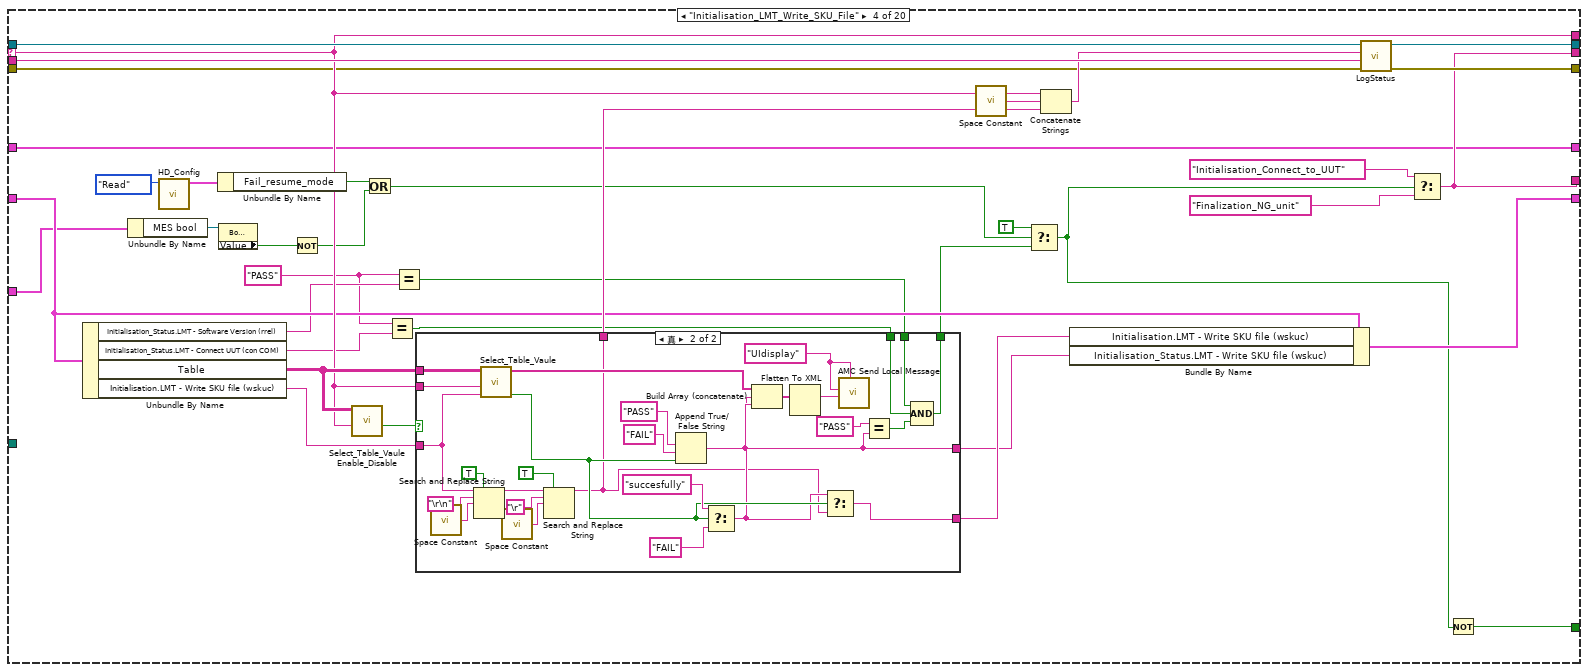
[diagram p6: hidden frame]
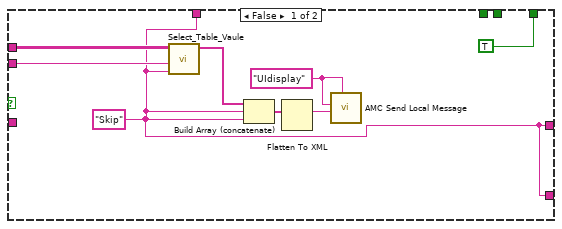
[diagram p7: hidden frame]
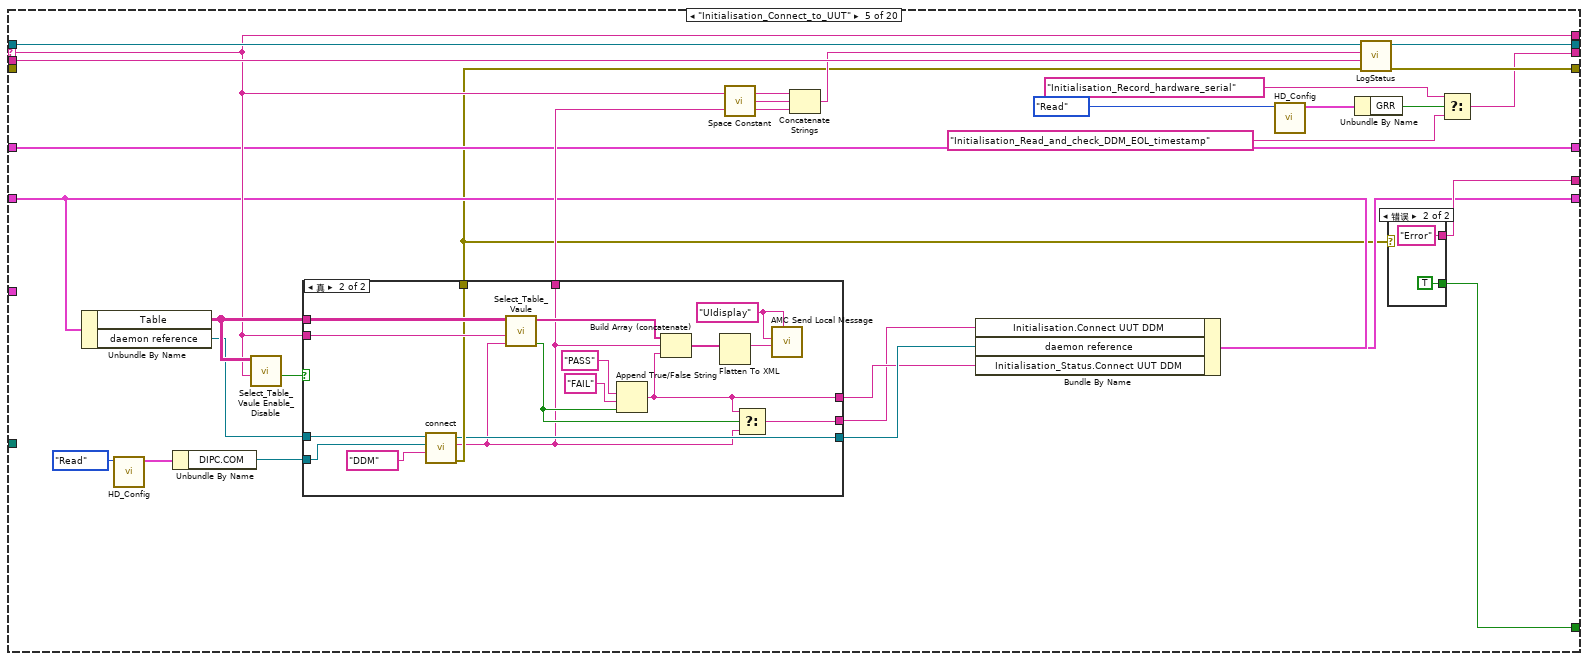
[diagram p8: hidden frame]
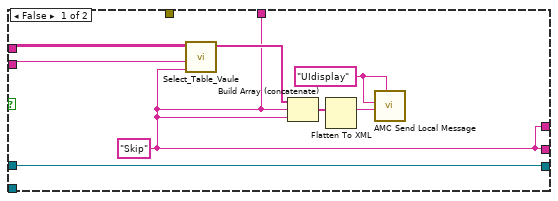
[diagram p10: hidden frame]
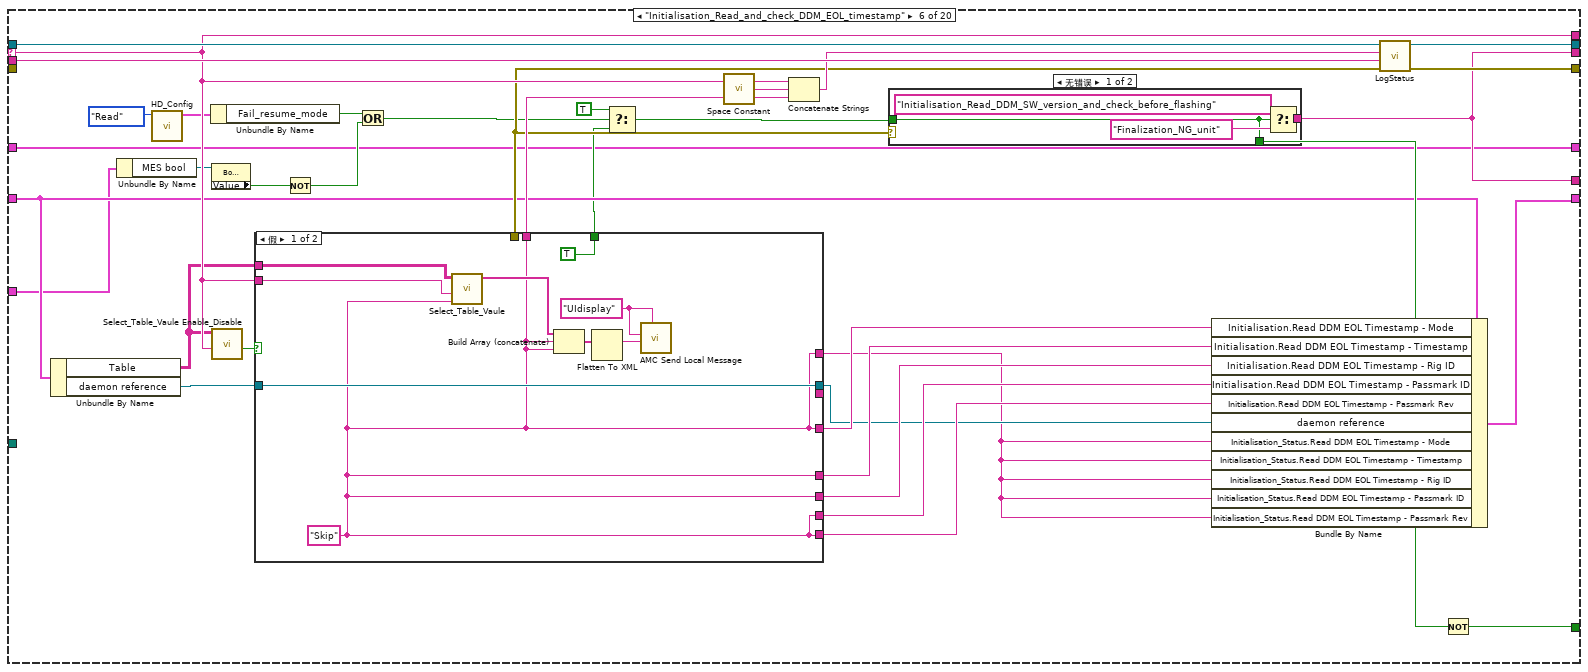
[diagram p11: hidden frame]
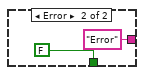
[diagram p12: hidden frame]
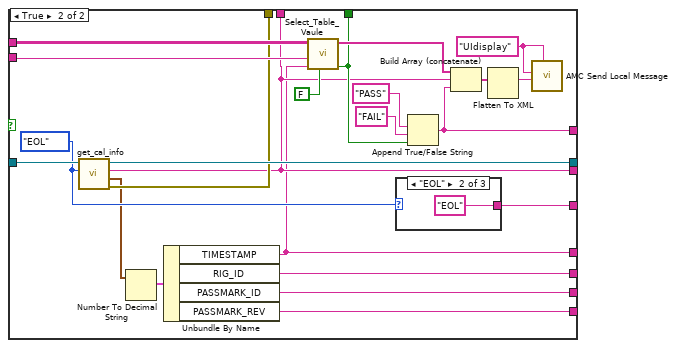
[diagram p13: hidden frame]
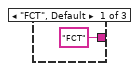
[diagram p14: hidden frame]
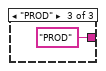
[diagram p15: hidden frame]
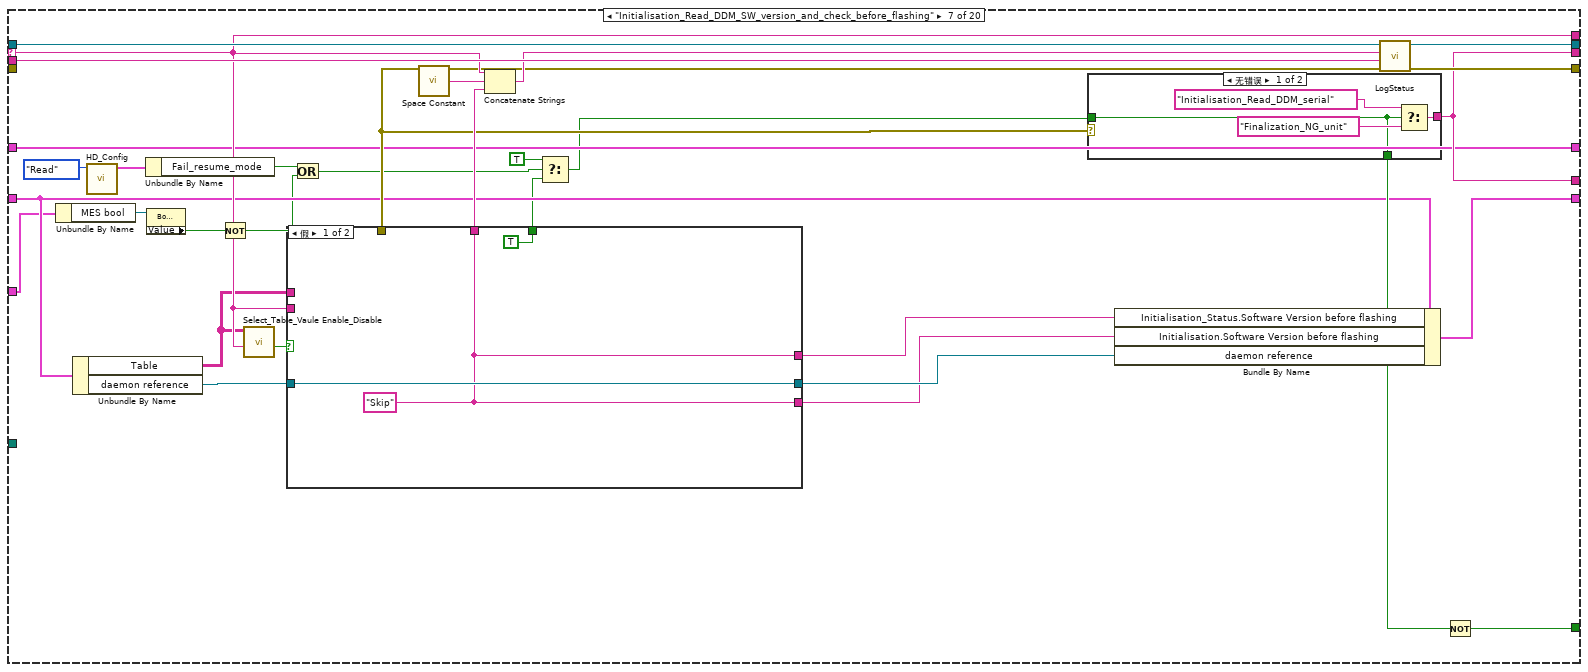
[diagram p16: hidden frame]
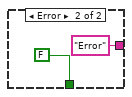
[diagram p17: hidden frame]
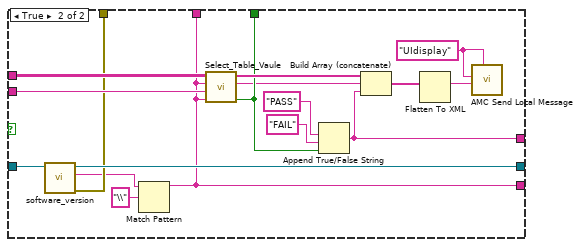
[diagram p18: hidden frame]
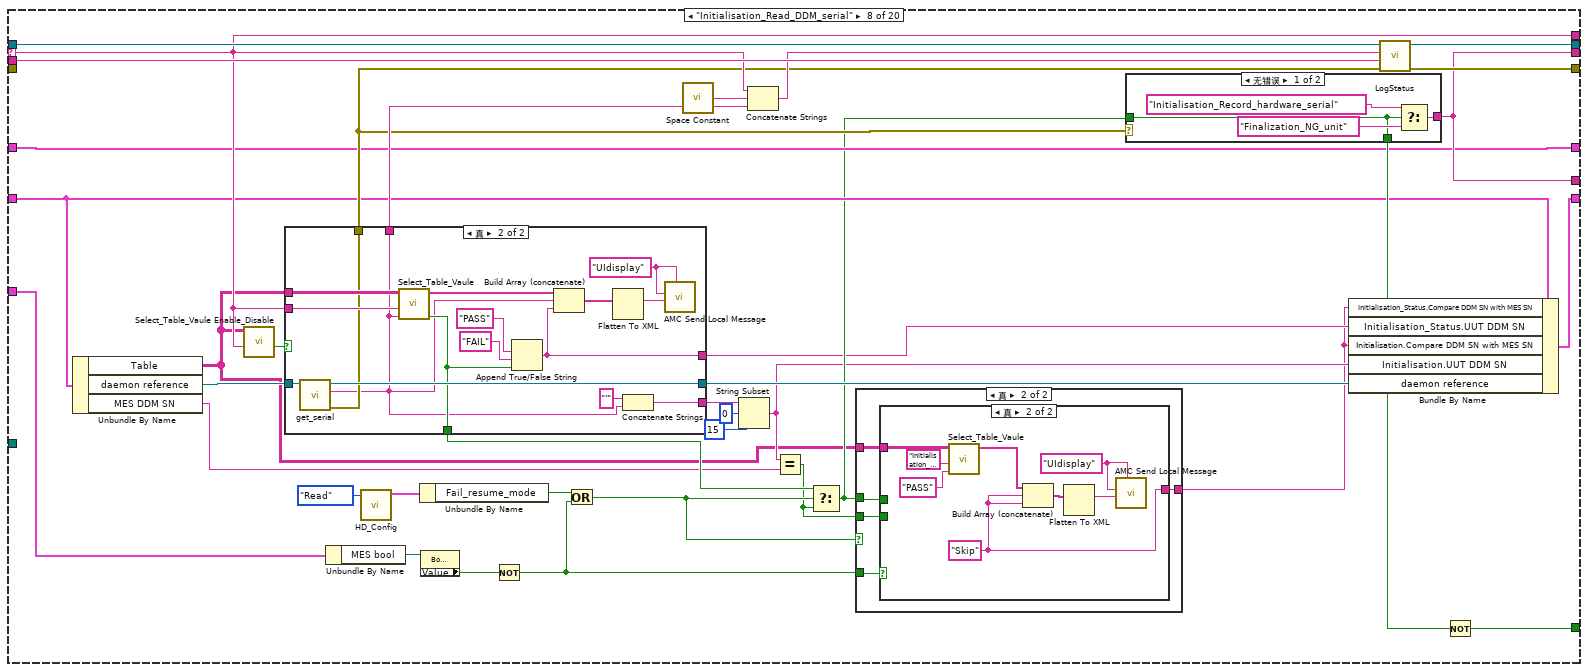
[diagram p19: hidden frame]
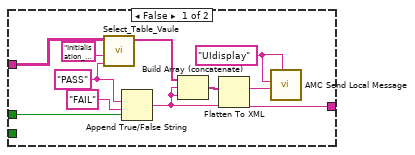
[diagram p20: hidden frame]
diagram:
  w7 = T5 {"Brush_ADC.bat"="Brush_ADC.bat", "Get Release Version.bat"="Get Release Version.bat", "Getting Software  Version.bat"="Getting Software  Version.bat", "Pump_ADC.bat"="Pump_ADC.bat", "Starting  Pump Motor.bat"="Starting  Pump Motor.bat", "Starting  Test Mode.bat"="Starting  Test Mode.bat", "Starting Brush Motor 1.bat"="Starting Brush Motor 1.bat", "Starting Brush Motor 2.bat"="Starting Brush Motor 2.bat", "Starting Brush Motor 3.bat"="Starting Brush Motor 3.bat", "Starting LED Test.bat"="Starting LED Test.bat", "Stopping  Brush Motor.bat"="Stopping  Brush Motor.bat", "Stopping  Pump Motor.bat"="Stopping  Pump Motor.bat", "Stopping  Test Mode.bat"="Stopping  Test Mode.bat", "1"="", "2"="", "3"="", "4"="", "5"="", "6"="", "7"="", "8"="", "9"="", "10"=""}  # .batCMD
  (unwired) string[] ["5.3.1_1 Set DC Power Supply", "5.3.1_2 Measure current from DC Power Supply", "5.3.2_1 Send Get VP and SC Version", "5.3.2_2 Stop Get VP and SC Version", "5.3.3_1 Starting LED Test", "5.3.3_2 Operator to manually judge each LED", "5.3.4_1 Self test", "5.3.4_3 GetResponse", "5.3.5_1 Connect dummy brush motor to UUT", "5.3.5_2 Starting Brush Motor in intensity 3", "5.3.5_3 Measure current consumption from DMM; Intensity 3", "5.3.5_4 Starting Brush Motor in intensity 2", "5.3.5_5 Measure current consumption from DMM; Intensity 2", "5.3.5_6 Starting Brush Motor in intensity 1", "5.3.5_7 Measure current consumption from DMM; Intensity 1", "5.3.5_8 Stopping Brush Motor", "5.3.6_1 Connect dummy pump motor to UUT", "5.3.6_2 Starting Pump Motor", "5.3.6_3 Measure current consumption from DMM", "5.3.6_4 Stopping Pump Motor", "5.3.7_1 MAC Address reading"] ("subarray")
  # "Starting Self Test.bat"
  # "5.3.5 Brush Motor Test"
  n1 = Unbundle By Name(w7) -> ()  [unwired: 13 out]
  n2 = call "1-BasePath.vi"("Step"=enum16{"Initial", "Write", "Read"}."Read") -> ("Path Out"=w4:path)  [unwired: 9 in, 1 out]
  n3 = Build Path(base path=w4, name or relative path="Tool") -> (appended path=w3:path)
  n4 = Build Path(base path=w3, name or relative path="Starting Self Test.bat") -> (appended path=w1:path)
  n5 = Flush Queue(queue="Message Queue out") -> (queue out=w13:T4)  [unwired: 1 in, 2 out]
  n6 = call "AMC Send Local Message.vi"("error in (no error)"="error in (no error)", "Message Name"="5.3.4_1 Self test", "Message Queue in"=w13) -> ("error out"=w18:errorcluster, "Message Queue out"=w19:T4)  [unwired: 7 in]
  n7 = while {
    tunnel: w19 -> [w52]
    tunnel: [w48] -> w12
    tunnel: w18 -> [w46]
    tunnel: [w43] -> w11
    shift-right: [w39] -> w15
    shift-left: "?" -> [w40]
    tunnel: [w35] -> w14
    tunnel: "AllControls In" -> [w28]
    shift-right: [w26] -> w8
    shift-left: "Data in" -> [w27]
    tunnel: w1 -> [w22]
    stop <- w31 stop-if-true
    n8 = Wait (ms)(milliseconds to wait=u32 1 ("等待时间（毫秒）")) -> ()  [unwired: 1 out]
    n9 = call "AMC Read Next Message.vi"("error in (no error)"=w46, "timeout (1ms)"=100, "Message Queue in"=w52) -> ("error out"=w45:errorcluster, "Message Value"=w37:string, "Message Name"=w50:string, "Message Queue out"=w51:T4)  [unwired: 1 in, 4 out]
    n10 = case shown="\"5.3.4_3 GetResponse\"" w50 {
      selector: w50 -> [_ w72 w116 w174 w236 w299 w370 w431 w514 w551 w601 w654 w759 w815 w879 w932 w994 w1086 w1171 w1231]
      tunnel: w51 -> [w56 w77 w121 w180 w244 w306 w378 w439 w521 w558 w608 w660 w766 w821 w885 w938 w1001 w1094 w1180 w1245]
      tunnel: [w56 w77 w121 w180 w244 w306 w378 w439 w521 w558 w608 w660 w766 w821 w885 w938 w1001 w1094 w1180 w1221] -> w49
      tunnel: w45 -> [w55 w71 w115 w173 _ _ _ _ _ w557 _ _ _ _ _ _ _ w1093 w1179 w1248]
      tunnel: [w55 w76 w120 w179 w243 w305 w377 w438 w520 w556 w607 w659 w765 w820 w884 w937 w1000 w1092 w1178 w1246] -> w44
      tunnel: [_ FALSE ("GRR") TRUE ("GRR") w169 w230 w297 w367 w429 w510 _ w597 w644 w754 w810 w874 w922 w988 _ TRUE w1227] -> w32
      tunnel: w40 -> [w54 w67 w111 w164 w227 w273 w361 w423 w505 w548 w575 w636 w738 w803 w856 w924 w981 w1076 w1159 w1232]
      tunnel: [w54 w67 w111 w164 w227 w273 w361 w423 w505 w548 w575 w636 w738 w803 w856 w924 w980 w1075 w1175 w1243] -> w39
      tunnel: w37 -> [_ w75 w119 w178 w242 w304 w376 w437 w519 w555 w606 w658 w764 w819 w883 w936 w999 w1091 w1177 w1247]
      tunnel: [_ w72 w116 w174 w236 w299 w370 w431 w514 w551 w601 w654 w759 w815 w879 w932 w994 w1086 w1171 w1231] -> w36
      tunnel: [_ "5.3.4_3 GetResponse" "5.3.5 Brush Motor Test" w171 w220 w296 w368 w430 w500 w544 "Initialisation_Flash_SW_follow_SKU" w648 w755 w798 w875 w919 "Initialisation_Get_and_check_Tester_Parameter" "Initialisation_Calculate_and_check_tester_parameter" w1161 w1228] -> w38
      tunnel: [_ _ _ w171 w232 w296 w368 w430 w511 _ w596 w645 w755 w811 w875 w919 w989 _ w1161 w1228] -> w35
      tunnel: w28 -> [_ _ _ w159 _ w276 w354 w417 _ _ _ w643 w741 _ w861 _ _ _ w1144 _]
      tunnel: w27 -> [w53 w66 w110 w163 w229 w291 w364 w426 w509 w541 w579 w640 w753 w807 w871 w923 w986 w1081 w1155 w1219]
      tunnel: [w53 w65 w109 w162 w228 w293 w363 w425 w506 w541 w578 w639 w751 w804 w870 w926 w983 w1078 w1153 w1220] -> w26
      tunnel: w22 -> [_ w59 w103 _ _ _ _ _ _ _ _ _ _ _ _ _ _ _ _ _]
      frame "假", Default {
      }
      frame "5.3.4_1 Self test" {
        n11 = Unbundle By Name(w66) -> ("Table"=w73:string[][], "OK/NG"=w62:bool)
        n12 = call "SendCmd_Tool.vi"("path_bat"=w59) -> ("return code"=w57:i32, "Led Test"=w58:string)  [unwired: 6 in, 7 out]
        n13 = call "Select_Table_Vaule Enable_Disable.vi"("Action"=w72, "Table"=w73) -> ("Enable"=w69:bool)  [unwired: 8 in, 1 out]
        n14 = case shown="真" w69 {
          tunnel: [w78 w92] -> w70
          tunnel: w73 -> [w80 w94]
          tunnel: w72 -> [w79 w93]
          tunnel: w58 -> [_ w92]
          tunnel: [w78 w91] -> w64
          tunnel: w62 -> [_ w90]
          tunnel: [_ w89] -> w61
          tunnel: w57 -> [_ w88]
          frame False {
            w84 = "UIdisplay" ("Process (\"\" - local)")
            w78 = "Skip" ("Action")
            n15 = call "Select_Table_Vaule.vi"("Vaule"=w78, "Action"=w79, "Table"=w80) -> ("vaule"=w81:string[])  [unwired: 7 in, 1 out]
            n16 = Build Array (concatenate)(w81, w78, w78) -> (w83:string[])
            n17 = Flatten To XML(anything=w83) -> (xml string=w82:string)
            n18 = call "AMC Send Local Message.vi"("Process (\"\" - local)"=w84, "Message Value"=w82, "Message Name"=w84) -> ()  [unwired: 7 in, 2 out]
          }
          frame True {
            w99 = "UIdisplay" ("Process (\"\" - local)")
            n19 = Equal To 0?(x=w88) -> (x = 0?=w87:bool)
            n20 = call "Select_Table_Vaule.vi"("Vaule"=w92, "Action"=w93, "Table"=w94) -> ("Result"=w85:bool, "vaule"=w100:string[])  [unwired: 7 in]
            n21 = And(x=w85, y=w87) -> (x .and. y?=w86:bool)
            n22 = Append True/False String(1:w86, 2:"FAIL" ("真字符串"), 3:"PASS" ("真字符串")) -> (0:w91:string)  [unwired: 1 in]
            n23 = Build Array (concatenate)(w100, w92, w91) -> (w98:string[])
            n24 = And(x=w86, y=w90) -> (x .and. y?=w89:bool)
            n25 = Flatten To XML(anything=w98) -> (xml string=w97:string)
            n26 = call "AMC Send Local Message.vi"("Process (\"\" - local)"=w99, "Message Value"=w97, "Message Name"=w99) -> ()  [unwired: 7 in, 2 out]
          }
        }
        n27 = Bundle By Name(cluster=w66, "Initialisation_Status.LMT - Connect UUT (con COM)"=w64, "OK/NG"=w61) -> (w65:T1)
        n28 = Concatenate Strings(w72, " :", w70) -> (w74:string)
        n29 = call "LogStatus.vi"("error in (no error)"=w71, "last message"=w75, "message"=w74) -> ("error  out"=w76:errorcluster)  [unwired: 8 in]
      }
      frame "5.3.4_3 GetResponse" {
        n30 = Unbundle By Name(w110) -> ("Table"=w117:string[][], "OK/NG"=w106:bool)
        n31 = call "SendCmd_Tool.vi"("path_bat"=w103) -> ("return code"=w102:i32, "Led Test"=w101:string)  [unwired: 6 in, 7 out]
        n32 = call "Select_Table_Vaule Enable_Disable.vi"("Action"=w116, "Table"=w117) -> ("Enable"=w113:bool)  [unwired: 8 in, 1 out]
        n33 = case shown="真" w113 {
          tunnel: [w122 w136] -> w114
          tunnel: w117 -> [w124 w138]
          tunnel: w116 -> [w123 w137]
          tunnel: w101 -> [_ w136]
          tunnel: [w122 w135] -> w108
          tunnel: w106 -> [_ w134]
          tunnel: [_ w133] -> w105
          tunnel: w102 -> [_ w132]
          frame False {
            w128 = "UIdisplay" ("Process (\"\" - local)")
            w122 = "Skip" ("Action")
            n34 = call "Select_Table_Vaule.vi"("Vaule"=w122, "Action"=w123, "Table"=w124) -> ("vaule"=w125:string[])  [unwired: 7 in, 1 out]
            n35 = Build Array (concatenate)(w125, w122, w122) -> (w127:string[])
            n36 = Flatten To XML(anything=w127) -> (xml string=w126:string)
            n37 = call "AMC Send Local Message.vi"("Process (\"\" - local)"=w128, "Message Value"=w126, "Message Name"=w128) -> ()  [unwired: 7 in, 2 out]
          }
          frame True {
            w143 = "UIdisplay" ("Process (\"\" - local)")
            n38 = Equal To 0?(x=w132) -> (x = 0?=w130:bool)
            n39 = call "Select_Table_Vaule.vi"("Vaule"=w136, "Action"=w137, "Table"=w138) -> ("Result"=w131:bool, "vaule"=w144:string[])  [unwired: 7 in]
            n40 = And(x=w131, y=w130) -> (x .and. y?=w129:bool)
            n41 = Append True/False String(1:w129, 2:"FAIL" ("真字符串"), 3:"PASS" ("真字符串")) -> (0:w135:string)  [unwired: 1 in]
            n42 = And(x=w129, y=w134) -> (x .and. y?=w133:bool)
            n43 = Build Array (concatenate)(w144, w136, w135) -> (w142:string[])
            n44 = Flatten To XML(anything=w142) -> (xml string=w141:string)
            n45 = call "AMC Send Local Message.vi"("Process (\"\" - local)"=w143, "Message Value"=w141, "Message Name"=w143) -> ()  [unwired: 7 in, 2 out]
          }
        }
        n46 = Bundle By Name(cluster=w110, "Initialisation_Status.LMT - Connect UUT (con COM)"=w108, "OK/NG"=w105) -> (w109:T1)
        n47 = Concatenate Strings(w116, " :", w114) -> (w118:string)
        n48 = call "LogStatus.vi"("error in (no error)"=w115, "last message"=w119, "message"=w118) -> ("error  out"=w120:errorcluster)  [unwired: 8 in]
      }
      frame "Initialisation_LMT_Write_SKU_File" {
        w151 = "PASS" ("真字符串")
        n49 = Unbundle By Name(w163) -> ("Initialisation_Status.LMT - Software Version (rrel)"=w153:string, "Initialisation_Status.LMT - Connect UUT (con COM)"=w152:string, "Table"=w175:string[][], "Initialisation.LMT - Write SKU file (wskuc)"=w166:string)
        n50 = Unbundle By Name(w159) -> ("MES bool"=w158:refnum<vi>)
        n51 = call "HD_Config.vi"("Step"=enum16{"Initial", "Write", "Read"}."Read") -> ("HD Config out"=w160:T11)  [unwired: 9 in, 1 out]
        n52 = Unbundle By Name(w160) -> ("Fail_resume_mode"=w157:bool)
        n53 = property class="Bool (严格)"(reference=w158) -> ("Value"=w156:bool)  [unwired: 1 in, 2 out]
        n54 = Not(x=w156) -> (.not. x?=w155:bool)
        n55 = call "Select_Table_Vaule Enable_Disable.vi"("Action"=w174, "Table"=w175) -> ("Enable"=w167:bool)  [unwired: 8 in, 1 out]
        n56 = Or(x=w157, y=w155) -> (x .or. y?=w148:bool)
        n57 = Equal?(x=w151, y=w152) -> (x = y?=w146:bool)
        n58 = Equal?(x=w151, y=w153) -> (x = y?=w147:bool)
        n59 = case shown="真" w167 {
          tunnel: [w181 w195] -> w168
          tunnel: w175 -> [w183 w210]
          tunnel: w174 -> [w182 w209]
          tunnel: w166 -> [_ w200]
          tunnel: [w181 w194] -> w165
          tunnel: [w181 w198] -> w150
          tunnel: w147 -> [_ w192]
          tunnel: w146 -> [_ w191]
          tunnel: [TRUE w189] -> w145
          frame False {
            w187 = "UIdisplay" ("Process (\"\" - local)")
            w181 = "Skip" ("Action")
            n60 = call "Select_Table_Vaule.vi"("Vaule"=w181, "Action"=w182, "Table"=w183) -> ("vaule"=w184:string[])  [unwired: 7 in, 1 out]
            n61 = Build Array (concatenate)(w184, w181, w181) -> (w186:string[])
            n62 = Flatten To XML(anything=w186) -> (xml string=w185:string)
            n63 = call "AMC Send Local Message.vi"("Process (\"\" - local)"=w187, "Message Value"=w185, "Message Name"=w187) -> ()  [unwired: 7 in, 2 out]
          }
          frame True {
            w215 = "UIdisplay" ("Process (\"\" - local)")
            n64 = call <vilib>:"Space Constant.vi"() -> ("String"=w206:string)
            n65 = Search and Replace String(replace all?=TRUE ("replace all? (F)"), input string=w200, search string="\r\n", replace string=w206) -> (result string=w208:string)  [unwired: 4 in, 3 out]
            n66 = call "Select_Table_Vaule.vi"("Vaule"=w200, "Action"=w209, "Table"=w210) -> ("Result"=w197:bool, "vaule"=w216:string[])  [unwired: 7 in]
            n67 = call <vilib>:"Space Constant.vi"() -> ("String"=w207:string)
            n68 = Search and Replace String(replace all?=TRUE ("replace all? (F)"), input string=w208, search string="\r", replace string=w207) -> (result string=w195:string)  [unwired: 4 in, 3 out]
            n69 = Append True/False String(1:w197, 2:"FAIL" ("真字符串"), 3:"PASS" ("真字符串")) -> (0:w198:string)  [unwired: 1 in]
            n70 = Select(t="succesfully" ("真字符串"), s=w197, f="FAIL" ("真字符串")) -> (s? t:f=w196:string)
            n71 = Build Array (concatenate)(w216, w196, w198) -> (w214:string[])
            n72 = Flatten To XML(anything=w214) -> (xml string=w213:string)
            n73 = Select(t=w196, s=w197, f=w195) -> (s? t:f=w194:string)
            n74 = call "AMC Send Local Message.vi"("Process (\"\" - local)"=w215, "Message Value"=w213, "Message Name"=w215) -> ()  [unwired: 7 in, 2 out]
            n75 = Equal?(x="PASS" ("真字符串"), y=w198) -> (x = y?=w190:bool)
            n76 = Compound Arithmetic op=AND ("复合运算")(w192, w191, w190) -> (w189:bool)
          }
        }
        n77 = call <vilib>:"Space Constant.vi"() -> ("String"=w176:string)
        n78 = Select(t=TRUE, s=w148, f=w145) -> (s? t:f=w149:bool)
        n79 = Concatenate Strings(w174, w176, w168) -> (w177:string)
        n80 = Bundle By Name(cluster=w163, "Initialisation.LMT - Write SKU file (wskuc)"=w165, "Initialisation_Status.LMT - Write SKU file (wskuc)"=w150) -> (w162:T1)
        n81 = call "LogStatus.vi"("error in (no error)"=w173, "last message"=w178, "message"=w177) -> ("error  out"=w179:errorcluster)  [unwired: 8 in]
        n82 = Select(t="Initialisation_Connect_to_UUT", s=w149, f="Finalization_NG_unit") -> (s? t:f=w171:string)
        n83 = Not(x=w149) -> (.not. x?=w169:bool)
      }
      frame "Initialisation_Connect_to_UUT" {
        n84 = Unbundle By Name(w229) -> ("Table"=w237:string[][], "daemon reference"=w231:refnum<k5>)
        n85 = call "HD_Config.vi"("Step"=enum16{"Initial", "Write", "Read"}."Read") -> ("HD Config out"=w233:T11)  [unwired: 9 in, 1 out]
        n86 = Unbundle By Name(w233) -> ("DIPC.COM"=w241:refnum<visa-resource-name>)
        n87 = call "Select_Table_Vaule Enable_Disable.vi"("Action"=w236, "Table"=w237) -> ("Enable"=w235:bool)  [unwired: 8 in, 1 out]
        n88 = case shown="真" w235 {
          tunnel: w241 -> [_ w271]
          tunnel: [w247 w256] -> w238
          tunnel: w237 -> [w249 w264]
          tunnel: w236 -> [w248 w263]
          tunnel: [_ w262] -> w225
          tunnel: w231 -> [w254 w260]
          tunnel: [w247 w257] -> w218
          tunnel: [w254 w259] -> w226
          tunnel: [w247 w255] -> w217
          frame False {
            w250 = "UIdisplay" ("Process (\"\" - local)")
            w247 = "Skip" ("response")
            n89 = call "Select_Table_Vaule.vi"("Vaule"=w247, "Action"=w248, "Table"=w249) -> ("vaule"=w253:string[])  [unwired: 7 in, 1 out]
            n90 = Build Array (concatenate)(w253, w247, w247) -> (w251:string[])
            n91 = Flatten To XML(anything=w251) -> (xml string=w252:string)
            n92 = call "AMC Send Local Message.vi"("Process (\"\" - local)"=w250, "Message Value"=w252, "Message Name"=w250) -> ()  [unwired: 7 in, 2 out]
          }
          frame True {
            w269 = "UIdisplay" ("Process (\"\" - local)")
            n93 = call "connect.vi"("Target"=T6 "DDM", "physical connection"=w271, "daemon reference in"=w260) -> ("error out"=w262:errorcluster, "response"=w256:string, "daemon reference out"=w259:refnum<k5>)  [unwired: 4 in, 2 out]
            n94 = call "Select_Table_Vaule.vi"("Vaule"=w256, "Action"=w263, "Table"=w264) -> ("Result"=w258:bool, "vaule"=w270:string[])  [unwired: 7 in]
            n95 = Append True/False String(1:w258, 2:"FAIL" ("真字符串"), 3:"PASS" ("真字符串")) -> (0:w257:string)  [unwired: 1 in]
            n96 = Build Array (concatenate)(w270, w256, w257) -> (w268:string[])
            n97 = Flatten To XML(anything=w268) -> (xml string=w267:string)
            n98 = Select(t=w257, s=w258, f=w256) -> (s? t:f=w255:string)
            n99 = call "AMC Send Local Message.vi"("Process (\"\" - local)"=w269, "Message Value"=w267, "Message Name"=w269) -> ()  [unwired: 7 in, 2 out]
          }
        }
        n100 = call <vilib>:"Space Constant.vi"() -> ("String"=w239:string)
        n101 = Concatenate Strings(w236, w239, w238) -> (w240:string)
        n102 = Bundle By Name(cluster=w229, "Initialisation.Connect UUT DDM"=w217, "daemon reference"=w226, "Initialisation_Status.Connect UUT DDM"=w218) -> (w228:T1)
        n103 = call "HD_Config.vi"("Step"=enum16{"Initial", "Write", "Read"}."Read") -> ("HD Config out"=w224:T11)  [unwired: 9 in, 1 out]
        n104 = Unbundle By Name(w224) -> ("GRR"=w222:bool)
        n105 = call "LogStatus.vi"("error in (no error)"=w225, "last message"=w242, "message"=w240) -> ("error  out"=w243:errorcluster)  [unwired: 8 in]
        n106 = case shown="错误" w225 {
          tunnel: [_ TRUE] -> w230
          tunnel: [_ "Error"] -> w232
          frame No Error {
          }
          frame Error {
          }
        }
        n107 = Select(t="Initialisation_Record_hardware_serial", s=w222, f="Initialisation_Read_and_check_DDM_EOL_timestamp") -> (s? t:f=w220:string)
      }
      frame "Initialisation_Read_and_check_DDM_EOL_timestamp" {
        n108 = Unbundle By Name(w291) -> ("Table"=w298:string[][], "daemon reference"=w303:refnum<k5>)
        n109 = Unbundle By Name(w276) -> ("MES bool"=w282:refnum<vi>)
        n110 = call "HD_Config.vi"("Step"=enum16{"Initial", "Write", "Read"}."Read") -> ("HD Config out"=w283:T11)  [unwired: 9 in, 1 out]
        n111 = Unbundle By Name(w283) -> ("Fail_resume_mode"=w281:bool)
        n112 = property class="Bool (严格)"(reference=w282) -> ("Value"=w280:bool)  [unwired: 1 in, 2 out]
        n113 = call "Select_Table_Vaule Enable_Disable.vi"("Action"=w299, "Table"=w298) -> ("Enable"=w300:bool)  [unwired: 8 in, 1 out]
        n114 = case shown="假" w300 {
          tunnel: w303 -> [w320 w344]
          tunnel: [TRUE w332] -> w275
          tunnel: [w320 w338] -> w285
          tunnel: [w313 w331] -> w294
          tunnel: w299 -> [w314 w337]
          tunnel: w298 -> [w315 w336]
          tunnel: [_ w334] -> w292
          tunnel: [_ w331] -> _
          tunnel: [w313 w330] -> w272
          tunnel: [w313 w329] -> w290
          tunnel: [w313 w325] -> w289
          tunnel: [w313 w324] -> w288
          tunnel: [w313 w323] -> w287
          tunnel: [w313 w322] -> w286
          frame False {
            w316 = "UIdisplay" ("Process (\"\" - local)")
            w313 = "Skip" ("response")
            n115 = call "Select_Table_Vaule.vi"("Vaule"=w313, "Action"=w314, "Table"=w315) -> ("vaule"=w319:string[])  [unwired: 7 in, 1 out]
            n116 = Build Array (concatenate)(w319, w313, w313) -> (w317:string[])
            n117 = Flatten To XML(anything=w317) -> (xml string=w318:string)
            n118 = call "AMC Send Local Message.vi"("Process (\"\" - local)"=w316, "Message Value"=w318, "Message Name"=w316) -> ()  [unwired: 7 in, 2 out]
          }
          frame True {
            w343 = "UIdisplay" ("Process (\"\" - local)")
            w328 = device_mode."EOL" ("Mode")
            n119 = call "get_cal_info.vi"("Mode"=w328, "daemon reference in"=w344) -> ("error out"=w334:errorcluster, "Parameter"=w327:T13, "response"=w331:string, "daemon reference out"=w338:refnum<k5>)  [unwired: 5 in, 1 out]
            n120 = Number To Decimal String(number=w327) -> (decimal integer string=w326:T14)  [unwired: 1 in]
            n121 = Unbundle By Name(w326) -> ("TIMESTAMP"=w325:string, "RIG_ID"=w324:string, "PASSMARK_ID"=w323:string, "PASSMARK_REV"=w322:string)
            n122 = call "Select_Table_Vaule.vi"("Boolean"=FALSE, "Vaule"=w325, "Action"=w337, "Table"=w336) -> ("Result"=w332:bool, "vaule"=w335:string[])  [unwired: 6 in]
            n123 = case shown="\"EOL\"" w328 {
              tunnel: ["FCT" ("Initialisation.5.3.2.8 Read DDM EOL Timestamp - Mode.Vaule") "EOL" ("Initialisation.5.3.2.8 Read DDM EOL Timestamp - Mode.Vaule") "PROD" ("Initialisation.5.3.2.8 Read DDM EOL Timestamp - Mode.Vaule")] -> w329
              frame "FCT", Default {
              }
              frame "EOL" {
              }
              frame "PROD" {
              }
            }
            n124 = Append True/False String(1:w332, 2:"FAIL" ("真字符串"), 3:"PASS" ("真字符串")) -> (0:w330:string)  [unwired: 1 in]
            n125 = Build Array (concatenate)(w335, w331, w330) -> (w342:string[])
            n126 = Flatten To XML(anything=w342) -> (xml string=w341:string)
            n127 = call "AMC Send Local Message.vi"("Process (\"\" - local)"=w343, "Message Value"=w341, "Message Name"=w343) -> ()  [unwired: 7 in, 2 out]
          }
        }
        n128 = Not(x=w280) -> (.not. x?=w278:bool)
        n129 = Or(x=w281, y=w278) -> (x .or. y?=w279:bool)
        n130 = Select(t=TRUE, s=w279, f=w275) -> (s? t:f=w274:bool)
        n131 = call <vilib>:"Space Constant.vi"() -> ("String"=w302:string)
        n132 = Concatenate Strings(w299, w302, w294) -> (w301:string)
        n133 = case shown="无错误" w292 {
          tunnel: w274 -> [w307 _]
          tunnel: [w308 "Error"] -> w296
          tunnel: [w307 FALSE] -> w295
          frame No Error {
            n134 = Select(t="Initialisation_Read_DDM_SW_version_and_check_before_flashing", s=w307, f="Finalization_NG_unit") -> (s? t:f=w308:string)
          }
          frame Error {
          }
        }
        n135 = Bundle By Name(cluster=w291, "Initialisation.Read DDM EOL Timestamp - Mode"=w290, "Initialisation.Read DDM EOL Timestamp - Timestamp"=w289, "Initialisation.Read DDM EOL Timestamp - Rig ID"=w288, "Initialisation.Read DDM EOL Timestamp - Passmark ID"=w287, "Initialisation.Read DDM EOL Timestamp - Passmark Rev"=w286, "daemon reference"=w285, "Initialisation_Status.Read DDM EOL Timestamp - Mode"=w272, "Initialisation_Status.Read DDM EOL Timestamp - Timestamp"=w272, "Initialisation_Status.Read DDM EOL Timestamp - Rig ID"=w272, "Initialisation_Status.Read DDM EOL Timestamp - Passmark ID"=w272, "Initialisation_Status.Read DDM EOL Timestamp - Passmark Rev"=w272) -> (w293:T1)
        n136 = call "LogStatus.vi"("error in (no error)"=w292, "last message"=w304, "message"=w301) -> ("error  out"=w305:errorcluster)  [unwired: 8 in]
        n137 = Not(x=w295) -> (.not. x?=w297:bool)
      }
      frame "Initialisation_Read_DDM_SW_version_and_check_before_flashing" {
        n138 = Unbundle By Name(w354) -> ("MES bool"=w358:refnum<vi>)
        n139 = Unbundle By Name(w364) -> ("Table"=w369:string[][], "daemon reference"=w375:refnum<k5>)
        n140 = call "HD_Config.vi"("Step"=enum16{"Initial", "Write", "Read"}."Read") -> ("HD Config out"=w359:T11)  [unwired: 9 in, 1 out]
        n141 = Unbundle By Name(w359) -> ("Fail_resume_mode"=w357:bool)
        n142 = property class="Bool (严格)"(reference=w358) -> ("Value"=w356:bool)  [unwired: 1 in, 2 out]
        n143 = Not(x=w356) -> (.not. x?=w355:bool)
        n144 = call "Select_Table_Vaule Enable_Disable.vi"("Action"=w370, "Table"=w369) -> ("Enable"=w371:bool)  [unwired: 8 in, 1 out]
        n145 = case shown="假" w371 {
          tunnel: w375 -> [w386 w398]
          tunnel: [TRUE w393] -> w351
          tunnel: [w386 w397] -> w362
          tunnel: [w385 w389] -> w372
          tunnel: w370 -> [_ w396]
          tunnel: w369 -> [_ w395]
          tunnel: [w385 w389] -> w349
          tunnel: [_ w392] -> w365
          tunnel: [w385 w388] -> w348
          frame False {
            w385 = "Skip" ("software string")
          }
          frame True {
            w403 = "UIdisplay" ("Process (\"\" - local)")
            n146 = call "software_version.vi"("daemon reference in"=w398) -> ("error out"=w392:errorcluster, "software string"=w391:string, "daemon reference out"=w397:refnum<k5>)  [unwired: 7 in, 1 out]
            n147 = Match Pattern(string=w391, regular expression="\\") -> (before substring=w389:string)  [unwired: 1 in, 3 out]
            n148 = call "Select_Table_Vaule.vi"("Vaule"=w389, "Action"=w396, "Table"=w395) -> ("Result"=w393:bool, "vaule"=w394:string[])  [unwired: 7 in]
            n149 = Append True/False String(1:w393, 2:"FAIL" ("真字符串"), 3:"PASS" ("真字符串")) -> (0:w388:string)  [unwired: 1 in]
            n150 = Build Array (concatenate)(w394, w389, w388) -> (w402:string[])
            n151 = Flatten To XML(anything=w402) -> (xml string=w401:string)
            n152 = call "AMC Send Local Message.vi"("Process (\"\" - local)"=w403, "Message Value"=w401, "Message Name"=w403) -> ()  [unwired: 7 in, 2 out]
          }
        }
        n153 = Or(x=w357, y=w355) -> (x .or. y?=w352:bool)
        n154 = call <vilib>:"Space Constant.vi"() -> ("String"=w374:string)
        n155 = Concatenate Strings(w370, w374, w372) -> (w373:string)
        n156 = Select(t=TRUE, s=w352, f=w351) -> (s? t:f=w350:bool)
        n157 = case shown="无错误" w365 {
          tunnel: [w381 "Error"] -> w368
          tunnel: w350 -> [w380 _]
          tunnel: [w380 FALSE ("Result")] -> w366
          frame No Error {
            n158 = Select(t="Initialisation_Read_DDM_serial" ("f"), s=w380, f="Finalization_NG_unit") -> (s? t:f=w381:string)
          }
          frame Error {
          }
        }
        n159 = Bundle By Name(cluster=w364, "Initialisation_Status.Software Version before flashing"=w348, "Initialisation.Software Version before flashing"=w349, "daemon reference"=w362) -> (w363:T1)
        n160 = call "LogStatus.vi"("error in (no error)"=w365, "last message"=w376, "message"=w373) -> ("error  out"=w377:errorcluster)  [unwired: 8 in]
        n161 = Not(x=w366) -> (.not. x?=w367:bool)
      }
      frame "Initialisation_Read_DDM_serial" {
        n162 = Unbundle By Name(w426) -> ("Table"=w406:string[][], "daemon reference"=w436:refnum<k5>, "MES DDM SN"=w413:string)
        n163 = call "Select_Table_Vaule Enable_Disable.vi"("Action"=w431, "Table"=w406) -> ("Enable"=w432:bool)  [unwired: 8 in, 1 out]
        n164 = case shown="真" w432 {
          tunnel: w436 -> [w480 w491]
          tunnel: [w480 w490] -> w424
          tunnel: [w479 w481] -> w433
          tunnel: w431 -> [_ w489]
          tunnel: w406 -> [_ w488]
          tunnel: [w479 w483] -> w410
          tunnel: [_ w486] -> w427
          tunnel: [w479 w485] -> w408
          tunnel: [_ w484] -> w414
          frame False {
            w479 = "Skip" ("software string")
          }
          frame True {
            w496 = "UIdisplay" ("Process (\"\" - local)")
            n165 = call "get_serial.vi"("daemon reference in"=w491) -> ("error out"=w486:errorcluster, "response"=w481:string, "daemon reference out"=w490:refnum<k5>)  [unwired: 7 in, 1 out]
            n166 = call "Select_Table_Vaule.vi"("Vaule"=w481, "Action"=w489, "Table"=w488) -> ("Result"=w484:bool, "vaule"=w487:string[])  [unwired: 7 in]
            n167 = Append True/False String(1:w484, 2:"FAIL" ("真字符串"), 3:"PASS" ("真字符串")) -> (0:w485:string)  [unwired: 1 in]
            n168 = Build Array (concatenate)(w487, w481, w485) -> (w495:string[])
            n169 = Flatten To XML(anything=w495) -> (xml string=w494:string)
            n170 = Concatenate Strings("'" ("字符串"), w481) -> (w483:string)
            n171 = call "AMC Send Local Message.vi"("Process (\"\" - local)"=w496, "Message Value"=w494, "Message Name"=w496) -> ()  [unwired: 7 in, 2 out]
          }
        }
        n172 = Unbundle By Name(w417) -> ("MES bool"=w420:refnum<vi>)
        n173 = call "HD_Config.vi"("Step"=enum16{"Initial", "Write", "Read"}."Read") -> ("HD Config out"=w421:T11)  [unwired: 9 in, 1 out]
        n174 = Unbundle By Name(w421) -> ("Fail_resume_mode"=w419:bool)
        n175 = property class="Bool (严格)"(reference=w420) -> ("Value"=w422:bool)  [unwired: 1 in, 2 out]
        n176 = Not(x=w422) -> (.not. x?=w405:bool)
        n177 = Or(x=w419, y=w405) -> (x .or. y?=w415:bool)
        n178 = call <vilib>:"Space Constant.vi"() -> ("String"=w435:string)
        n179 = String Subset(string=w410, offset (0)=0 ("偏移量(0)"), length (rest)=15 ("长度（剩余）")) -> (substring=w409:string)
        n180 = Concatenate Strings(w431, w435, w433) -> (w434:string)
        n181 = Equal?(x=w409, y=w413) -> (x = y?=w404:bool)
        n182 = Select(t=w414, s=w415, f=w404) -> (s? t:f=w416:bool)
        n183 = case shown="真" w415 {
          tunnel: [w440 w454] -> w407
          tunnel: w416 -> [w448 w451]
          tunnel: w406 -> [w443 w452]
          tunnel: w405 -> [_ w453]
          tunnel: w404 -> [_ w450]
          frame False {
            w447 = "UIdisplay" ("Process (\"\" - local)")
            w441 = "PASS" ("真字符串")
            n184 = call "Select_Table_Vaule.vi"("Vaule"=w441, "Action"="Initialisation_Compare_DDM_serial_MES_SN", "Table"=w443) -> ("vaule"=w444:string[])  [unwired: 7 in, 1 out]
            n185 = Append True/False String(1:w448, 2:"FAIL" ("真字符串"), 3:w441) -> (0:w440:string)  [unwired: 1 in]
            n186 = Build Array (concatenate)(w444, w440, w440) -> (w446:string[])
            n187 = Flatten To XML(anything=w446) -> (xml string=w445:string)
            n188 = call "AMC Send Local Message.vi"("Process (\"\" - local)"=w447, "Message Value"=w445, "Message Name"=w447) -> ()  [unwired: 7 in, 2 out]
          }
          frame True {
            n189 = case shown="真" w453 {
              tunnel: [w456 w465] -> w454
              tunnel: w452 -> [w457 w466]
              tunnel: w451 -> [_ _]
              tunnel: w450 -> [w455 _]
              frame False {
                w463 = "UIdisplay" ("Process (\"\" - local)")
                w458 = "PASS" ("真字符串")
                n190 = call "Select_Table_Vaule.vi"("Vaule"=w458, "Action"="Initialisation_Compare_DDM_serial_MES_SN", "Table"=w457) -> ("vaule"=w460:string[])  [unwired: 7 in, 1 out]
                n191 = Append True/False String(1:w455, 2:"FAIL" ("真字符串"), 3:w458) -> (0:w456:string)  [unwired: 1 in]
                n192 = Build Array (concatenate)(w460, w456, w456) -> (w462:string[])
                n193 = Flatten To XML(anything=w462) -> (xml string=w461:string)
                n194 = call "AMC Send Local Message.vi"("Process (\"\" - local)"=w463, "Message Value"=w461, "Message Name"=w463) -> ()  [unwired: 7 in, 2 out]
              }
              frame True {
                w472 = "UIdisplay" ("Process (\"\" - local)")
                w465 = "Skip" ("output string")
                n195 = call "Select_Table_Vaule.vi"("Vaule"="PASS" ("真字符串"), "Action"="Initialisation_Compare_DDM_serial_MES_SN", "Table"=w466) -> ("vaule"=w469:string[])  [unwired: 7 in, 1 out]
                n196 = Build Array (concatenate)(w469, w465, w465) -> (w471:string[])
                n197 = Flatten To XML(anything=w471) -> (xml string=w470:string)
                n198 = call "AMC Send Local Message.vi"("Process (\"\" - local)"=w472, "Message Value"=w470, "Message Name"=w472) -> ()  [unwired: 7 in, 2 out]
              }
            }
          }
        }
        n199 = case shown="无错误" w427 {
          tunnel: [w474 "Error"] -> w430
          tunnel: w416 -> [w473 _]
          tunnel: [w473 FALSE ("Result")] -> w428
          frame No Error {
            n200 = Select(t="Initialisation_Record_hardware_serial", s=w473, f="Finalization_NG_unit") -> (s? t:f=w474:string)
          }
          frame Error {
          }
        }
        n201 = Bundle By Name(cluster=w426, "Initialisation_Status.Compare DDM SN with MES SN"=w407, "Initialisation_Status.UUT DDM SN"=w408, "Initialisation.Compare DDM SN with MES SN"=w407, "Initialisation.UUT DDM SN"=w409, "daemon reference"=w424) -> (w425:T1)
        n202 = call "LogStatus.vi"("error in (no error)"=w427, "last message"=w437, "message"=w434) -> ("error  out"=w438:errorcluster)  [unwired: 8 in]
        n203 = Not(x=w428) -> (.not. x?=w429:bool)
      }
      frame "Initialisation_Record_hardware_serial" {
        n204 = Unbundle By Name(w509) -> ("Table"=w513:string[][], "daemon reference"=w518:refnum<k5>)
        n205 = call "Select_Table_Vaule Enable_Disable.vi"("Action"=w514, "Table"=w513) -> ("Enable"=w512:bool)  [unwired: 8 in, 1 out]
        n206 = case shown="假" w512 {
          tunnel: w518 -> [w525 w535]
          tunnel: [w525 w534] -> w507
          tunnel: [w524 w529] -> w515
          tunnel: w514 -> [_ w533]
          tunnel: w513 -> [_ w532]
          tunnel: [w524 w528] -> w498
          tunnel: [_ w527] -> w508
          tunnel: [w524 w526] -> w497
          frame False {
            w524 = "Skip" ("software string")
            (unwired) TRUE
          }
          frame True {
            w540 = "UIdisplay" ("Process (\"\" - local)")
            n207 = call "hardware_serial.vi"("daemon reference in"=w535) -> ("error out"=w527:errorcluster, "hardware_serial"=w528:string, "response"=w529:string, "daemon reference out"=w534:refnum<k5>)  [unwired: 6 in, 1 out]
            n208 = call "Select_Table_Vaule.vi"("Vaule"=w529, "Action"=w533, "Table"=w532) -> ("Result"=w530:bool, "vaule"=w531:string[])  [unwired: 7 in]
            n209 = Append True/False String(1:w530, 2:"FAIL" ("真字符串"), 3:"PASS" ("真字符串")) -> (0:w526:string)  [unwired: 1 in]
            n210 = Build Array (concatenate)(w531, w529, w526) -> (w539:string[])
            n211 = Flatten To XML(anything=w539) -> (xml string=w538:string)
            n212 = call "AMC Send Local Message.vi"("Process (\"\" - local)"=w540, "Message Value"=w538, "Message Name"=w540) -> ()  [unwired: 7 in, 2 out]
          }
        }
        n213 = call <vilib>:"Space Constant.vi"() -> ("String"=w517:string)
        n214 = Concatenate Strings(w514, w517, w515) -> (w516:string)
        n215 = Bundle By Name(cluster=w509, "Initialisation_Status.Read Hardware Serial"=w497, "Initialisation.Read Hardware Serial"=w498, "daemon reference"=w507) -> (w506:T1)
        n216 = call "HD_Config.vi"("Step"=enum16{"Initial", "Write", "Read"}."Read") -> ("HD Config out"=w504:T11)  [unwired: 9 in, 1 out]
        n217 = Unbundle By Name(w504) -> ("GRR"=w502:bool)
        n218 = call "LogStatus.vi"("error in (no error)"=w508, "last message"=w519, "message"=w516) -> ("error  out"=w520:errorcluster)  [unwired: 8 in]
        n219 = case shown="错误" w508 {
          tunnel: [_ TRUE] -> w510
          tunnel: [_ "Error"] -> w511
          frame No Error {
          }
          frame Error {
          }
        }
        n220 = Select(t="Initialisation_Read_DDM_SW_Version_and_check_after_flashing", s=w502, f="Initialisation_search_backup_folder_before_flashing_and_check_file_is_exist") -> (s? t:f=w500:string)
      }
      frame "Initialisation_search_backup_folder_before_flashing_and_check_file_is_exist" {
        n221 = Unbundle By Name(w541) -> ("Table"=w550:string[][], "Config"=w543:string[][], "Initialisation.Read Hardware Serial"=w542:string)
        n222 = call "Select_Table_Vaule Enable_Disable.vi"("Action"=w551, "Table"=w550) -> ("Enable"=w549:bool)  [unwired: 8 in, 1 out]
        n223 = case shown="假" w549 {
          tunnel: ["Skip" ("software string") w566] -> w552
          tunnel: w551 -> [_ _]
          tunnel: w550 -> [_ _]
          tunnel: [TRUE ("file or folder exists?") w561] -> w547
          tunnel: w543 -> [_ _]
          tunnel: w542 -> [_ w562]
          frame False {
          }
          frame True {
            n224 = call "PathChoose.vi"(11:PathChoose."backup_before_flashing") -> ("Path_Out"=w564:path)  [unwired: 10 in]
            n225 = List Folder(path=w564) -> (filenames=w563:string[])  [unwired: 3 in, 3 out]
            n226 = for {
              tunnel: w563 -> [w572] mode=indexing
              tunnel: w562 -> [w571]
              tunnel: [w569] -> w561
              stop <- w569 stop-if-true
              n227 = Search and Replace String(input string=w572, search string=w571) -> (number of replacements=w570:i32)  [unwired: 6 in, 3 out]
              n228 = Greater Than 0?(x=w570) -> (x > 0?=w569:bool)
            }
            n229 = Append True/False String(1:w561, 2:"non exist" ("false string"), 3:"exist" ("true string")) -> (0:w566:string)  [unwired: 1 in]
          }
        }
        n230 = call <vilib>:"Space Constant.vi"() -> ("String"=w554:string)
        n231 = Concatenate Strings(w551, w554, w552) -> (w553:string)
        n232 = call "LogStatus.vi"("error in (no error)"=w557, "last message"=w555, "message"=w553) -> ("error  out"=w556:errorcluster)  [unwired: 8 in]
        n233 = Select(t="Initialisation_Flash_SW_follow_SKU", s=w547, f="Initialisation_Backup_DDM_NVM") -> (s? t:f=w544:string)
      }
      frame "Initialisation_Backup_DDM_NVM" {
        n234 = Unbundle By Name(w579) -> ("Table"=w600:string[][], "daemon reference"=w605:refnum<k5>, "Config"=w598:string[][], "Initialisation.Read Hardware Serial"=w581:string)
        n235 = call "PathChoose.vi"(11:PathChoose."backup_before_flashing") -> ("Path_Out"=w588:path)  [unwired: 10 in]
        n236 = Path To String(path=w588) -> (string=w589:string)
        n237 = Format Date/Time String(time format string (%c)="%Y%m%d%H%M%S" ("时间格式字符串(%c)")) -> (date/time string=w590:string)  [unwired: 2 in]
        n238 = call "Select_Table_Vaule Enable_Disable.vi"("Action"=w601, "Table"=w600) -> ("Enable"=w599:bool)  [unwired: 8 in, 1 out]
        n239 = Concatenate Strings(w589, "\\" ("字符串"), w581, "_" ("string"), w590, ".json" ("string")) -> (w587:string)
        n240 = String To Path(string=w587) -> (path=w594:path)
        n241 = call <vilib>:"Check if File or Folder Exists.vi"("path"=w594) -> ("error out"=w592:errorcluster, "file or folder exists?"=w593:bool, "dup path"=w591:path)  [unwired: 8 in]
        n242 = case shown="假" w593 {
          tunnel: w592 -> [w612 w613]
          tunnel: w591 -> [w609 w614]
          tunnel: [w609 w614] -> w580
          tunnel: [w611 w613] -> _
          frame False {
            n243 = Open/Create/Replace File(file path (use dialog)=w609, error in=w612, operation (0:open)=T8."create") -> (error out=w611:errorcluster)  [unwired: 3 in, 2 out]
          }
          frame True {
          }
        }
        n244 = case shown="假" w599 {
          tunnel: w605 -> [w618 w629]
          tunnel: [w618 w628] -> w576
          tunnel: [w617 w619] -> w577
          tunnel: w601 -> [_ w627]
          tunnel: w600 -> [_ w626]
          tunnel: w598 -> [_ _]
          tunnel: [_ w622] -> w595
          tunnel: w580 -> [_ w621]
          tunnel: [w617 w620] -> w573
          tunnel: [w617 w619] -> w574
          frame False {
            w617 = "Skip" ("software string")
            (unwired) TRUE
          }
          frame True {
            w634 = "UIdisplay" ("Process (\"\" - local)")
            n245 = call "backup_nvm.vi"("type"=read_nvm_section."CAL", "File Path"=w621, "daemon reference in"=w629) -> ("error out"=w622:errorcluster, "response"=w619:string, "daemon reference out"=w628:refnum<k5>)  [unwired: 5 in, 1 out]
            n246 = call "Select_Table_Vaule.vi"("Vaule"=w619, "Action"=w627, "Table"=w626) -> ("Result"=w624:bool, "vaule"=w625:string[])  [unwired: 7 in]
            n247 = Append True/False String(1:w624, 2:"FAIL" ("真字符串"), 3:"PASS" ("真字符串")) -> (0:w620:string)  [unwired: 1 in]
            n248 = Build Array (concatenate)(w625, w619, w620) -> (w633:string[])
            n249 = Flatten To XML(anything=w633) -> (xml string=w632:string)
            n250 = call "AMC Send Local Message.vi"("Process (\"\" - local)"=w634, "Message Value"=w632, "Message Name"=w634) -> ()  [unwired: 7 in, 2 out]
          }
        }
        n251 = call <vilib>:"Space Constant.vi"() -> ("String"=w604:string)
        n252 = Concatenate Strings(w601, w604, w577) -> (w603:string)
        n253 = Bundle By Name(cluster=w579, "Initialisation_Status.Backup PCBA Calibration EEPROM Response - CAL"=w573, "Initialisation.Backup PCBA Calibration EEPROM Response - CAL"=w574, "daemon reference"=w576) -> (w578:T1)
        n254 = call "LogStatus.vi"("error in (no error)"=w595, "last message"=w606, "message"=w603) -> ("error  out"=w607:errorcluster)  [unwired: 8 in]
        n255 = case shown="错误" w595 {
          tunnel: [_ TRUE] -> w597
          tunnel: [_ "Error"] -> w596
          frame No Error {
          }
          frame Error {
          }
        }
      }
      frame "Initialisation_Flash_SW_follow_SKU" {
        n256 = Unbundle By Name(w640) -> ("Table"=w653:string[][], "daemon reference"=w657:refnum<k5>, "Config"=w651:string[][])
        n257 = Unbundle By Name(w643) -> ("MainVI"=w642:refnum<vi>)
        n258 = call "Select_Table_Vaule Enable_Disable.vi"("Action"=w654, "Table"=w653) -> ("Enable"=w652:bool)  [unwired: 8 in, 1 out]
        n259 = case shown="真" w652 {
          tunnel: w657 -> [w665 w694]
          tunnel: [w665 w693] -> w638
          tunnel: [w663 w666] -> w641
          tunnel: w654 -> [_ w692]
          tunnel: w653 -> [_ w691]
          tunnel: w651 -> [_ w688]
          tunnel: [TRUE w689] -> w647
          tunnel: string[] ["Initialisation_DDM_Firmware_Hex", "Initialisation_DDM_Firmware_bin", "Initialisation_Flashing_wait_time", "Initialisation_Flashing_Mode", "Initialisation_Product_Mode"] -> [_ w687]
          tunnel: [_ w677] -> w637
          tunnel: w642 -> [_ w675]
          tunnel: [w663 w671] -> w635
          tunnel: [_ w670] -> _
          tunnel: [_ w666] -> _
          tunnel: [_ w668] -> _
          tunnel: [_ w666] -> _
          frame False {
            w663 = "Skip" ("software string")
          }
          frame True {
            w699 = "UIdisplay" ("Process (\"\" - local)")
            n260 = for {
              tunnel: w688 -> [w733]
              tunnel: w687 -> [w732] mode=indexing
              tunnel: [w731] -> w686 mode=indexing
              n261 = call "Index_Config.vi"("Action"=w732, "config"=w733) -> ("data"=w731:string)  [unwired: 9 in]
            }
            n262 = call <vilib>:"Set Busy.vi"("VI reference (current VI)"=w675) -> ("error out"=w676:errorcluster)  [unwired: 9 in, 1 out]
            n263 = Index Array(array=w686) -> (element #1=w685:string, element #2=w667:string, element #3=w670:string, element #4=w672:string, element #5=w673:string)  [unwired: 5 in]
            n264 = String To Path(string=w685) -> (path=w684:path)
            n265 = String To Path(string=w667) -> (path=w683:path)
            n266 = Decimal String To Number(string=w670) -> (number=w682:i32)  [unwired: 2 in, 1 out]
            n267 = Multiply(x=w682, y=1000) -> (x*y=w680:i32)
            n268 = case shown="\"EVT3\", 默认" w673 {
              tunnel: w694 -> [w706 w730]
              tunnel: [w707 w729] -> w693
              tunnel: w684 -> [_ w727]
              tunnel: w683 -> [w705 w726]
              tunnel: w680 -> [w703 w725]
              tunnel: [w704 w724] -> w678
              tunnel: [w701 w723] -> w677
              tunnel: w676 -> [w702 w722]
              tunnel: w672 -> [w700 _]
              frame "EVT3", Default {
                n269 = case shown="\"SPC\", 默认" w700 {
                  tunnel: [w713 w721] -> w707
                  tunnel: w706 -> [w714 w720]
                  tunnel: w705 -> [w709 w719]
                  tunnel: [w712 w718] -> w704
                  tunnel: w703 -> [w708 w717]
                  tunnel: w702 -> [w710 w716]
                  tunnel: [w711 w715] -> w701
                  frame "SPC", Default {
                    n270 = call "set_product_config_bin.vi"("timeout (25000ms)"=w708, "error in (no error)"=w710, "firmware image bin file"=w709, "daemon reference in"=w714) -> ("error out"=w711:errorcluster, "response"=w712:string, "daemon reference out"=w713:refnum<k5>)  [unwired: 4 in, 1 out]
                  }
                  frame "FF" {
                    n271 = call "flash_firmware_bin.vi"("timeout (25000ms)"=w717, "error in (no error)"=w716, "firmware path"=w719, "daemon reference in"=w720) -> ("error out"=w715:errorcluster, "response"=w718:string, "daemon reference out"=w721:refnum<k5>)  [unwired: 4 in, 1 out]
                  }
                }
              }
              frame "EVT2" {
                n272 = call "flash_firmware.vi"("timeout (25000ms)"=w725, "SW 4.1 and above?"=TRUE, "error in (no error)"=w722, "SIV bin path"=w726, "firmware path"=w727, "daemon reference in"=w730) -> ("error out"=w723:errorcluster, "response"=w724:string, "daemon reference out"=w729:refnum<k5>)  [unwired: 2 in, 1 out]
              }
            }
            n273 = Match Pattern(string=w667, regular expression="data\\") -> (after substring=w668:string)  [unwired: 1 in, 3 out]
            n274 = Match Pattern(string=w678, regular expression="\\") -> (before substring=w666:string)  [unwired: 1 in, 3 out]
            n275 = call "Select_Table_Vaule.vi"("Vaule"=w666, "Action"=w692, "Table"=w691) -> ("Result"=w689:bool, "vaule"=w690:string[])  [unwired: 7 in]
            n276 = call <vilib>:"Unset Busy.vi"("error in (no error)"=w677, "VI reference (current VI)"=w675) -> ("error out"=w674:errorcluster)  [unwired: 9 in]
            n277 = call <vilib>:"Clear Errors.vi"("error in (no error)"=w674) -> ()  [unwired: 5 in, 2 out]
            n278 = Append True/False String(1:w689, 2:"FAIL" ("真字符串"), 3:"PASS" ("真字符串")) -> (0:w671:string)  [unwired: 1 in]
            n279 = Build Array (concatenate)(w690, w666, w671) -> (w698:string[])
            n280 = Flatten To XML(anything=w698) -> (xml string=w697:string)
            n281 = call "AMC Send Local Message.vi"("Process (\"\" - local)"=w699, "Message Value"=w697, "Message Name"=w699) -> ()  [unwired: 7 in, 2 out]
          }
        }
        n282 = call <vilib>:"Space Constant.vi"() -> ("String"=w656:string)
        n283 = Concatenate Strings(w654, w656, w641) -> (w655:string)
        n284 = Bundle By Name(cluster=w640, "daemon reference"=w638, "Initialisation.Flash Firmware Version"=w635, "Initialisation_Status.Flash Firmware Version"=w635) -> (w639:T1)
        n285 = call "LogStatus.vi"("error in (no error)"=w637, "last message"=w658, "message"=w655) -> ("error  out"=w659:errorcluster)  [unwired: 8 in]
        n286 = Select(t="Initialisation_Read_DDM_SW_Version_and_check_after_flashing", s=w647, f="Reflashing") -> (s? t:f=w648:string)
        n287 = case shown="错误" w637 {
          tunnel: [_ TRUE] -> w644
          tunnel: [_ "Error"] -> w645
          frame No Error {
          }
          frame Error {
          }
        }
      }
      frame "Initialisation_Read_DDM_SW_Version_and_check_after_flashing" {
        n288 = Unbundle By Name(w753) -> ("Table"=w758:string[][], "daemon reference"=w763:refnum<k5>, "Config"=w756:string[][])
        n289 = Unbundle By Name(w741) -> ("MES bool"=w744:refnum<vi>)
        n290 = call "HD_Config.vi"("Step"=enum16{"Initial", "Write", "Read"}."Read") -> ("HD Config out"=w743:T11)  [unwired: 9 in, 1 out]
        n291 = Unbundle By Name(w743) -> ("GRR"=w737:bool, "Fail_resume_mode"=w745:bool)
        n292 = property class="Bool (严格)"(reference=w744) -> ("Value"=w746:bool)  [unwired: 1 in, 2 out]
        n293 = call "Select_Table_Vaule Enable_Disable.vi"("Action"=w759, "Table"=w758) -> ("Enable"=w757:bool)  [unwired: 8 in, 1 out]
        n294 = Not(x=w746) -> (.not. x?=w747:bool)
        n295 = case shown="真" w757 {
          tunnel: w763 -> [w778 w786]
          tunnel: [w778 w785] -> w750
          tunnel: [w776 w780] -> w760
          tunnel: w759 -> [_ w789]
          tunnel: w758 -> [_ w788]
          tunnel: w756 -> [_ _]
          tunnel: [TRUE w784] -> w739
          tunnel: [w776 w780] -> w734
          tunnel: [_ w783] -> w752
          tunnel: [w776 w779] -> w735
          frame False {
            w776 = "Skip" ("software string")
          }
          frame True {
            w794 = "UIdisplay" ("Process (\"\" - local)")
            n296 = call "software_version.vi"("daemon reference in"=w786) -> ("error out"=w783:errorcluster, "software string"=w781:string, "daemon reference out"=w785:refnum<k5>)  [unwired: 7 in, 1 out]
            n297 = Match Pattern(string=w781, regular expression="\\") -> (before substring=w780:string)  [unwired: 1 in, 3 out]
            n298 = call "Select_Table_Vaule.vi"("Vaule"=w780, "Action"=w789, "Table"=w788) -> ("Result"=w784:bool, "vaule"=w787:string[])  [unwired: 7 in]
            n299 = Append True/False String(1:w784, 2:"FAIL" ("真字符串"), 3:"PASS" ("真字符串")) -> (0:w779:string)  [unwired: 1 in]
            n300 = Build Array (concatenate)(w787, w780, w779) -> (w793:string[])
            n301 = Flatten To XML(anything=w793) -> (xml string=w792:string)
            n302 = call "AMC Send Local Message.vi"("Process (\"\" - local)"=w794, "Message Value"=w792, "Message Name"=w794) -> ()  [unwired: 7 in, 2 out]
          }
        }
        n303 = Or(x=w745, y=w747) -> (x .or. y?=w749:bool)
        n304 = call <vilib>:"Space Constant.vi"() -> ("String"=w762:string)
        n305 = Select(t=TRUE, s=w749, f=w739) -> (s? t:f=w740:bool)
        n306 = Concatenate Strings(w759, w762, w760) -> (w761:string)
        n307 = case shown="无错误" w752 {
          tunnel: [w771 "Error"] -> w755
          tunnel: w740 -> [w767 _]
          tunnel: [w769 FALSE ("Result")] -> w736
          tunnel: w737 -> [w768 _]
          frame No Error {
            w770 = "Initialisation_Set_SKU_Config_base_on_variant"
            n308 = Select(t=w768, s=w768, f=w767) -> (s? t:f=w769:bool)
            n309 = Select(t=w770, s=w767, f="Finalization_NG_unit") -> (s? t:f=w772:string)
            n310 = Select(t=w770, s=w768, f=w772) -> (s? t:f=w771:string)
          }
          frame Error {
          }
        }
        n311 = Bundle By Name(cluster=w753, "daemon reference"=w750, "Initialisation.Check SW Version"=w734, "Initialisation.Read DDM SW Version after flashing"=w734, "Initialisation_Status.Check SW Version"=w735, "Initialisation_Status.Read DDM SW Version after flashing"=w735) -> (w751:T1)
        n312 = call "LogStatus.vi"("error in (no error)"=w752, "last message"=w764, "message"=w761) -> ("error  out"=w765:errorcluster)  [unwired: 8 in]
        n313 = Not(x=w736) -> (.not. x?=w754:bool)
      }
      frame "Initialisation_Set_SKU_Config_base_on_variant" {
        # "文件与LMT调用文件一样.mem文件"
        n314 = Unbundle By Name(w807) -> ("Table"=w814:string[][], "daemon reference"=w818:refnum<k5>, "Config"=w812:string[][])
        n315 = call "Select_Table_Vaule Enable_Disable.vi"("Action"=w815, "Table"=w814) -> ("Enable"=w813:bool)  [unwired: 8 in, 1 out]
        n316 = case shown="真" w813 {
          tunnel: w818 -> [w826 w841]
          tunnel: [w826 w840] -> w805
          tunnel: [w824 w830] -> w809
          tunnel: w815 -> [_ w845]
          tunnel: w814 -> [_ w844]
          tunnel: w812 -> [_ w839]
          tunnel: [TRUE w842] -> _
          tunnel: string[] ["Initialisation_SKU_Config_Hex", "Initialisation_SKU_ID"] -> [_ w837]
          tunnel: [_ w838] -> w806
          tunnel: [w824 w834] -> w795
          tunnel: [w824 w833] -> w796
          tunnel: [_ w831] -> _
          frame False {
            w824 = "Skip" ("software string")
          }
          frame True {
            w850 = "UIdisplay" ("Process (\"\" - local)")
            n317 = for {
              tunnel: w839 -> [w853]
              tunnel: w837 -> [w852] mode=indexing
              tunnel: [w851] -> w836 mode=indexing
              n318 = call "Index_Config.vi"("Action"=w852, "config"=w853) -> ("data"=w851:string)  [unwired: 9 in]
            }
            n319 = Index Array(array=w836) -> (element #1=w829:string, element #2=w831:string)  [unwired: 2 in]
            n320 = String To Path(string=w829) -> (path=w835:path)
            n321 = Match Pattern(string=w829, regular expression="data\\" ("正则表达式")) -> (after substring=w827:string)  [unwired: 1 in, 3 out]
            n322 = call "set_sku.vi"("SKU ID"=w831, "sku hex filepath"=w835, "daemon reference in"=w841) -> ("error out"=w838:errorcluster, "response"=w833:string, "daemon reference out"=w840:refnum<k5>)  [unwired: 5 in, 1 out]
            n323 = call <vilib>:"Space Constant.vi"() -> ("String"=w828:string)
            n324 = call "Select_Table_Vaule.vi"("Vaule"=w833, "Action"=w845, "Table"=w844) -> ("Result"=w842:bool, "vaule"=w843:string[])  [unwired: 7 in]
            n325 = Concatenate Strings(w827, w828, w833) -> (w830:string)
            n326 = Append True/False String(1:w842, 2:"FAIL" ("真字符串"), 3:"PASS" ("真字符串")) -> (0:w834:string)  [unwired: 1 in]
            n327 = Build Array (concatenate)(w843, w830, w834) -> (w849:string[])
            n328 = Flatten To XML(anything=w849) -> (xml string=w848:string)
            n329 = call "AMC Send Local Message.vi"("Process (\"\" - local)"=w850, "Message Value"=w848, "Message Name"=w850) -> ()  [unwired: 7 in, 2 out]
          }
        }
        n330 = call <vilib>:"Space Constant.vi"() -> ("String"=w817:string)
        n331 = Concatenate Strings(w815, w817, w809) -> (w816:string)
        n332 = Bundle By Name(cluster=w807, "Initialisation_Status.Set SKU Config"=w795, "Initialisation.Set SKU Config"=w796, "daemon reference"=w805) -> (w804:T1)
        n333 = call "HD_Config.vi"("Step"=enum16{"Initial", "Write", "Read"}."Read") -> ("HD Config out"=w800:T11)  [unwired: 9 in, 1 out]
        n334 = Unbundle By Name(w800) -> ("GRR"=w802:bool)
        n335 = call "LogStatus.vi"("error in (no error)"=w806, "last message"=w819, "message"=w816) -> ("error  out"=w820:errorcluster)  [unwired: 8 in]
        n336 = case shown="错误" w806 {
          tunnel: [_ TRUE] -> w810
          tunnel: [_ "Error"] -> w811
          frame No Error {
          }
          frame Error {
          }
        }
        n337 = Select(t="Initialisation_Set_DDM_to_EOL_Mode", s=w802, f="Initialisation_Get_and_check_UUT_Ready_Status") -> (s? t:f=w798:string)
      }
      frame "Initialisation_Get_and_check_UUT_Ready_Status" {
        n338 = Unbundle By Name(w871) -> ("Table"=w878:string[][], "daemon reference"=w882:refnum<k5>, "Config"=w876:string[][])
        n339 = Unbundle By Name(w861) -> ("MES bool"=w864:refnum<vi>)
        n340 = call "HD_Config.vi"("Step"=enum16{"Initial", "Write", "Read"}."Read") -> ("HD Config out"=w863:T11)  [unwired: 9 in, 1 out]
        n341 = Unbundle By Name(w863) -> ("Fail_resume_mode"=w865:bool)
        n342 = property class="Bool (严格)"(reference=w864) -> ("Value"=w866:bool)  [unwired: 1 in, 2 out]
        n343 = call "Select_Table_Vaule Enable_Disable.vi"("Action"=w879, "Table"=w878) -> ("Enable"=w877:bool)  [unwired: 8 in, 1 out]
        n344 = case shown="假" w877 {
          tunnel: w882 -> [w901 w906]
          tunnel: [w901 w905] -> w857
          tunnel: ["Skip" ("software string") w903] -> w872
          tunnel: w879 -> [w893 w910]
          tunnel: w878 -> [w894 w909]
          tunnel: w876 -> [_ _]
          tunnel: [TRUE w907] -> w859
          tunnel: [_ w904] -> w858
          tunnel: [w892 w903] -> w855
          tunnel: [w892 w902] -> w854
          frame False {
            w898 = "UIdisplay" ("Process (\"\" - local)")
            w892 = "Skip" ("Action")
            n345 = call "Select_Table_Vaule.vi"("Vaule"=w892, "Action"=w893, "Table"=w894) -> ("vaule"=w895:string[])  [unwired: 7 in, 1 out]
            n346 = Build Array (concatenate)(w895, w892, w892) -> (w897:string[])
            n347 = Flatten To XML(anything=w897) -> (xml string=w896:string)
            n348 = call "AMC Send Local Message.vi"("Process (\"\" - local)"=w898, "Message Value"=w896, "Message Name"=w898) -> ()  [unwired: 7 in, 2 out]
          }
          frame True {
            w915 = "UIdisplay" ("Process (\"\" - local)")
            n349 = call "ready_status.vi"("daemon reference in"=w906) -> ("error out"=w904:errorcluster, "response"=w903:string, "daemon reference out"=w905:refnum<k5>)  [unwired: 7 in, 1 out]
            n350 = call "Select_Table_Vaule.vi"("Vaule"=w903, "Action"=w910, "Table"=w909) -> ("Result"=w907:bool, "vaule"=w908:string[])  [unwired: 7 in]
            n351 = Append True/False String(1:w907, 2:"FAIL" ("真字符串"), 3:"PASS" ("真字符串")) -> (0:w902:string)  [unwired: 1 in]
            n352 = Build Array (concatenate)(w908, w903, w902) -> (w914:string[])
            n353 = Flatten To XML(anything=w914) -> (xml string=w913:string)
            n354 = call "AMC Send Local Message.vi"("Process (\"\" - local)"=w915, "Message Value"=w913, "Message Name"=w915) -> ()  [unwired: 7 in, 2 out]
          }
        }
        n355 = Not(x=w866) -> (.not. x?=w867:bool)
        n356 = Or(x=w865, y=w867) -> (x .or. y?=w869:bool)
        n357 = Select(t=TRUE, s=w869, f=w859) -> (s? t:f=w860:bool)
        n358 = call <vilib>:"Space Constant.vi"() -> ("String"=w881:string)
        n359 = Concatenate Strings(w879, w881, w872) -> (w880:string)
        n360 = case shown="无错误" w858 {
          tunnel: [w887 "Error"] -> w875
          tunnel: w860 -> [w886 _]
          tunnel: [w886 FALSE ("Result")] -> w873
          frame No Error {
            n361 = Select(t="Initialisation_Set_DDM_to_EOL_Mode", s=w886, f="Finalization_NG_unit") -> (s? t:f=w887:string)
          }
          frame Error {
          }
        }
        n362 = Bundle By Name(cluster=w871, "Initialisation_Status.Ready Status"=w854, "Initialisation.Ready Status"=w855, "daemon reference"=w857) -> (w870:T1)
        n363 = call "LogStatus.vi"("error in (no error)"=w858, "last message"=w883, "message"=w880) -> ("error  out"=w884:errorcluster)  [unwired: 8 in]
        n364 = Not(x=w873) -> (.not. x?=w874:bool)
      }
      frame "Initialisation_Set_DDM_to_EOL_Mode" {
        n365 = Unbundle By Name(w923) -> ("Table"=w931:string[][], "daemon reference"=w935:refnum<k5>, "Config"=w929:string[][])
        n366 = call "Select_Table_Vaule Enable_Disable.vi"("Action"=w932, "Table"=w931) -> ("Enable"=w930:bool)  [unwired: 8 in, 1 out]
        n367 = case shown="假" w930 {
          tunnel: w935 -> [w947 w954]
          tunnel: [w947 w953] -> w925
          tunnel: [w945 w951] -> w928
          tunnel: w932 -> [_ w958]
          tunnel: w931 -> [_ w957]
          tunnel: w929 -> [_ _]
          tunnel: [TRUE w955] -> _
          tunnel: [_ w952] -> w927
          tunnel: [_ w951] -> _
          tunnel: [w945 w950] -> w916
          tunnel: [w945 w948] -> w917
          frame False {
            w945 = "Skip" ("software string")
          }
          frame True {
            w949 = device_mode."EOL" ("Mode")
            w963 = "UIdisplay" ("Process (\"\" - local)")
            n368 = call "set_device_mode.vi"("Mode"=w949, "daemon reference in"=w954) -> ("error out"=w952:errorcluster, "response"=w951:string, "daemon reference out"=w953:refnum<k5>)  [unwired: 6 in, 1 out]
            n369 = call "Select_Table_Vaule.vi"("Vaule"=w951, "Action"=w958, "Table"=w957) -> ("Result"=w955:bool, "vaule"=w956:string[])  [unwired: 7 in]
            n370 = case shown="\"EOL\"" w949 {
              tunnel: ["FCT" ("Initialisation.5.3.2.8 Read DDM EOL Timestamp - Mode.Vaule") "EOL" ("Initialisation.5.3.2.8 Read DDM EOL Timestamp - Mode.Vaule") "PROD" ("Initialisation.5.3.2.8 Read DDM EOL Timestamp - Mode.Vaule")] -> w948
              frame "FCT", Default {
              }
              frame "EOL" {
              }
              frame "PROD" {
              }
            }
            n371 = call "Time Delay"("error in (no error)"=w952) -> ()  [unwired: 10 in, 1 out]
            n372 = Append True/False String(1:w955, 2:"FAIL" ("真字符串"), 3:"PASS" ("真字符串")) -> (0:w950:string)  [unwired: 1 in]
            n373 = Build Array (concatenate)(w956, w951, w950) -> (w962:string[])
            n374 = Flatten To XML(anything=w962) -> (xml string=w961:string)
            n375 = call "AMC Send Local Message.vi"("Process (\"\" - local)"=w963, "Message Value"=w961, "Message Name"=w963) -> ()  [unwired: 7 in, 2 out]
          }
        }
        n376 = call <vilib>:"Space Constant.vi"() -> ("String"=w934:string)
        n377 = Concatenate Strings(w932, w934, w928) -> (w933:string)
        n378 = call "HD_Config.vi"("Step"=enum16{"Initial", "Write", "Read"}."Read") -> ("HD Config out"=w921:T11)  [unwired: 9 in, 1 out]
        n379 = Unbundle By Name(w921) -> ("GRR"=w918:bool)
        n380 = case shown="无错误" w927 {
          tunnel: [w939 TRUE] -> w922
          tunnel: [w942 "Error"] -> w919
          tunnel: w918 -> [w939 _]
          frame No Error {
            n381 = Select(t="Power_Tunings_and_AW_Performance_Test", s=w939, f="Initialisation_Get_and_check_DDM_Parameter") -> (s? t:f=w942:string)
          }
          frame Error {
          }
        }
        n382 = Bundle By Name(cluster=w923, "Initialisation_Status.Set Device Mode to EOL"=w916, "Initialisation.Set Device Mode to EOL"=w917, "daemon reference"=w925) -> (w926:T1)
        n383 = call "LogStatus.vi"("error in (no error)"=w927, "last message"=w936, "message"=w933) -> ("error  out"=w937:errorcluster)  [unwired: 8 in]
      }
      frame "Initialisation_Get_and_check_DDM_Parameter" {
        n384 = Unbundle By Name(w986) -> ("Table"=w993:string[][], "daemon reference"=w998:refnum<k5>, "Config"=w991:string[][])
        n385 = call "Select_Table_Vaule Enable_Disable.vi"("Action"=w994, "Table"=w993) -> ("Enable"=w992:bool)  [unwired: 8 in, 1 out]
        n386 = case shown="真" w992 {
          tunnel: w998 -> [w1007 w1036]
          tunnel: [w1007 w1035] -> w972
          tunnel: [w1006 w1027] -> w995
          tunnel: w994 -> [_ w1033]
          tunnel: w993 -> [_ w1037]
          tunnel: w991 -> [_ _]
          tunnel: [_ w1026] -> w984
          tunnel: T10[] ["voltage", "current", "power", "speed", "pressure"] ("Parameter") -> [_ w1022]
          tunnel: [w1005 w1014] -> w985
          tunnel: [w1005 w1013] -> w982
          tunnel: [_ w1012] -> w979
          tunnel: [_ w1008] -> w978
          frame False {
            w1006 = "Skip" ("software string")
            n387 = Initialize Array(w1006, 5 ("维数大小")) -> (w1005:string[])
          }
          frame True {
            w1031 = string[] ["Initialisation_DDM_Voltage", "Initialisation_DDM_Current", "Initialisation_DDM_Power", "Initialisation_DDM_Speed", "Initialisation_DDM_Pressure"]
            n388 = for {
              tunnel: [w1043] -> w1021 mode=indexing
              tunnel: [w1042] -> w1026
              tunnel: [w1038] -> w1023 mode=indexing
              shift-right: [w1044] -> w1035
              shift-left: w1036 -> [w1045]
              tunnel: w1022 -> [w1039] mode=indexing
              n389 = Build Array(w1039) -> (w1040:T10[])
              n390 = call "get_parameter.vi"("Parameter"=w1040, "daemon reference in"=w1045) -> ("error out"=w1042:errorcluster, "response"=w1043:string, "values"=w1041:dbl[], "daemon reference out"=w1044:refnum<k5>)  [unwired: 5 in, 1 out]
              n391 = Index Array(array=w1041) -> (element=w1038:dbl)  [unwired: 1 in]
            }
            n392 = in-place {
              w1050 = 1000.0
              n393 = in-place-array #1(w1023, 3, 4) -> (w1049:dbl, w1046:dbl)
              n394 = Divide(x=w1049, y=w1050) -> (x/y=w1048:dbl)
              n395 = Divide(x=w1046, y=w1050) -> (x/y=w1047:dbl)
              n396 = in-place-array #1(w1048, w1047) -> (w1012:dbl[])  [unwired: 2 out]
            }
            n397 = Array To Spreadsheet String(delimiter (Tab)=",", array=w1021, 3:"" ("format string")) -> (spreadsheet string=w1020:string)
            n398 = Build Array (concatenate)(w1033, w1031) -> (w1034:string[])
            n399 = Number To Fractional String(number=w1012) -> (F-format string=w1013:string[])  [unwired: 3 in]
            n400 = Interleave 1D Arrays(w1031, w1013) -> (w1030:string[])
            n401 = Build Array (concatenate)(w1020, w1013) -> (w1032:string[])
            n402 = Array To Spreadsheet String(delimiter (Tab)=";" ("分隔符(Tab)"), array=w1030, 3:"" ("格式字符串")) -> (spreadsheet string=w1027:string)
            n403 = for {
              tunnel: w1037 -> [w1057]
              tunnel: w1032 -> [w1055] mode=indexing
              tunnel: w1034 -> [w1054] mode=indexing
              tunnel: [w1052] -> w1015 mode=indexing
              tunnel: [w1051] -> w1009 mode=indexing
              w1062 = "UIdisplay" ("Process (\"\" - local)")
              n404 = call "Select_Table_Vaule.vi"("Boolean"=TRUE, "Vaule"=w1055, "Action"=w1054, "Table"=w1057) -> ("Result"=w1051:bool, "vaule"=w1056:string[])  [unwired: 6 in]
              n405 = Append True/False String(1:w1051, 2:"FAIL" ("真字符串"), 3:"PASS" ("真字符串")) -> (0:w1052:string)  [unwired: 1 in]
              n406 = Build Array (concatenate)(w1056, w1055, w1052) -> (w1061:string[])
              n407 = Flatten To XML(anything=w1061) -> (xml string=w1060:string)
              n408 = call "AMC Send Local Message.vi"("Process (\"\" - local)"=w1062, "Message Value"=w1060, "Message Name"=w1062) -> ()  [unwired: 7 in, 2 out]
            }
            n409 = Delete From Array(array=w1009, length=1 ("长度"), index=0 ("索引")) -> (array with subset deleted=w1008:bool[])  [unwired: 1 out]
            n410 = Delete From Array(array=w1015, length=1 ("长度"), index=0 ("索引")) -> (array with subset deleted=w1014:string[])  [unwired: 1 out]
          }
        }
        n411 = call <vilib>:"Space Constant.vi"() -> ("String"=w997:string)
        n412 = Concatenate Strings(w994, w997, w995) -> (w996:string)
        n413 = Index Array(array=w982) -> (element #1=w973:string, element #2=w974:string, element #3=w975:string, element #4=w976:string, element #5=w977:string)  [unwired: 5 in]
        n414 = Index Array(array=w985) -> (element #1=w971:string, element #2=w970:string, element #3=w969:string, element #4=w968:string, element #5=w967:string)  [unwired: 5 in]
        n415 = Bundle By Name(cluster=w986, "daemon reference"=w972, "Initialisation.DDM Parameter - Voltage"=w973, "Initialisation.DDM Parameter - Current"=w974, "Initialisation.DDM Parameter - Power"=w975, "Initialisation.DDM Parameter - Speed"=w976, "Initialisation.DDM Parameter - Pressure"=w977, "Initialisation_Status.DDM Parameter - Voltage"=w971, "Initialisation_Status.DDM Parameter - Current"=w970, "Initialisation_Status.DDM Parameter - Power"=w969, "Initialisation_Status.DDM Parameter - Speed"=w968, "Initialisation_Status.DDM Parameter - Pressure"=w967) -> (w983:T1)
        n416 = Bundle By Name(cluster=w981, "Initialisation.DDM_Parameter"=w979, "Initialisation.DDM_Parameter_status"=w978) -> (w980:T3)
        n417 = call "LogStatus.vi"("error in (no error)"=w984, "last message"=w999, "message"=w996) -> ("error  out"=w1000:errorcluster)  [unwired: 8 in]
        n418 = case shown="错误" w984 {
          tunnel: [_ TRUE] -> w988
          tunnel: [_ "Error"] -> w989
          frame No Error {
          }
          frame Error {
          }
        }
      }
      frame "Initialisation_Get_and_check_Tester_Parameter" {
        n419 = Unbundle By Name(w1081) -> ("Table"=w1085:string[][], "daemon reference"=w1090:refnum<k5>, "Config"=w1083:string[][])
        n420 = call "Select_Table_Vaule Enable_Disable.vi"("Action"=w1086, "Table"=w1085) -> ("Enable"=w1084:bool)  [unwired: 8 in, 1 out]
        n421 = case shown="假" w1084 {
          tunnel: w1090 -> [w1098 w1120]
          tunnel: [w1098 w1120] -> w1079
          tunnel: [w1097 w1111] -> w1087
          tunnel: w1086 -> [_ w1118]
          tunnel: w1085 -> [_ w1121]
          tunnel: w1083 -> [_ _]
          tunnel: [w1096 w1110] -> w1077
          tunnel: [w1096 w1105] -> w1080
          tunnel: [_ w1104] -> _
          tunnel: [_ w1103] -> w1074
          tunnel: [_ w1099] -> w1073
          frame False {
            w1097 = "Skip" ("software string")
            n422 = Initialize Array(w1097, 5 ("维数大小")) -> (w1096:string[])
          }
          frame True {
            w1115 = string[] ["Initialisation_PM_Voltage", "Initialisation_PM_Current", "Initialisation_PM_Power", "Initialisation_Ambient_Pressure", "Initialisation_Ambient_Temperature", "Initialisation_Tester_Reference_Ambient_Pressure"]
            n423 = call "Initialisation_Tester_Parameter.vi"() -> ("Pressure(Pa)"=w1109:dbl, "Initialisation_Tester_Parameter"=w1103:dbl[])  [unwired: 10 in]
            n424 = Number To Fractional String(number=w1103) -> (F-format string=w1110:string[])  [unwired: 3 in]
            n425 = Number To Fractional String(number=w1109) -> (F-format string=w1104:string)  [unwired: 3 in]
            n426 = Interleave 1D Arrays(w1115, w1110) -> (w1114:string[])
            n427 = Array To Spreadsheet String(delimiter (Tab)=";" ("分隔符(Tab)"), array=w1114, 3:"" ("格式字符串")) -> (spreadsheet string=w1111:string)
            n428 = Build Array (concatenate)(w1118, w1115) -> (w1119:string[])
            n429 = Build Array (concatenate)("", w1110) -> (w1117:string[])
            n430 = for {
              tunnel: w1121 -> [w1128]
              tunnel: w1117 -> [w1126] mode=indexing
              tunnel: w1119 -> [w1125] mode=indexing
              tunnel: [w1123] -> w1108 mode=indexing
              tunnel: [w1122] -> w1100 mode=indexing
              w1133 = "UIdisplay" ("Process (\"\" - local)")
              n431 = call "Select_Table_Vaule.vi"("Boolean"=TRUE, "Vaule"=w1126, "Action"=w1125, "Table"=w1128) -> ("Result"=w1122:bool, "vaule"=w1127:string[])  [unwired: 6 in]
              n432 = Append True/False String(1:w1122, 2:"FAIL" ("真字符串"), 3:"PASS" ("真字符串")) -> (0:w1123:string)  [unwired: 1 in]
              n433 = Build Array (concatenate)(w1127, w1126, w1123) -> (w1132:string[])
              n434 = Flatten To XML(anything=w1132) -> (xml string=w1131:string)
              n435 = call "AMC Send Local Message.vi"("Process (\"\" - local)"=w1133, "Message Value"=w1131, "Message Name"=w1133) -> ()  [unwired: 7 in, 2 out]
            }
            n436 = Delete From Array(array=w1100, length=1 ("长度"), index=0 ("索引")) -> (array with subset deleted=w1099:bool[])  [unwired: 1 out]
            n437 = Delete From Array(array=w1108, length=1 ("长度"), index=0 ("索引")) -> (array with subset deleted=w1105:string[])  [unwired: 1 out]
          }
        }
        n438 = call <vilib>:"Space Constant.vi"() -> ("String"=w1089:string)
        n439 = Concatenate Strings(w1086, w1089, w1087) -> (w1088:string)
        n440 = Index Array(array=w1080) -> (element #1=w1067:string, element #2=w1066:string, element #3=w1065:string, element #4=w1064:string, element #5=w1063:string)  [unwired: 5 in]
        n441 = Index Array(array=w1077) -> (element #1=w1072:string, element #2=w1071:string, element #3=w1070:string, element #4=w1069:string, element #5=w1068:string)  [unwired: 5 in]
        n442 = Bundle By Name(cluster=w1081, "daemon reference"=w1079, "Initialisation.Tester Parameter - Voltage"=w1072, "Initialisation.Tester Parameter - Current"=w1071, "Initialisation.Tester Parameter - Power"=w1070, "Initialisation.Tester Parameter - Ambient Pressure"=w1069, "Initialisation.Tester Parameter - Ambient Temperature"=w1068, "Initialisation_Status.Tester Parameter - Voltage"=w1067, "Initialisation_Status.Tester Parameter - Current"=w1066, "Initialisation_Status.Tester Parameter - Power"=w1065, "Initialisation_Status.Tester Parameter - Ambient Pressure"=w1064, "Initialisation_Status.Tester Parameter - Ambient Temperature"=w1063) -> (w1078:T1)
        n443 = Bundle By Name(cluster=w1076, "Initialisation.Get_Tester_Parameter"=w1074, "Initialisation.Get_Tester_Parameter_status"=w1073) -> (w1075:T3)
        n444 = call "LogStatus.vi"("error in (no error)"=w1093, "last message"=w1091, "message"=w1088) -> ("error  out"=w1092:errorcluster)  [unwired: 8 in]
      }
      frame "Initialisation_Calculate_and_check_tester_parameter" {
        n445 = Unbundle By Name(w1159) -> ("Initialisation.DDM_Parameter"=w1158:dbl[], "Initialisation.Get_Tester_Parameter"=w1157:dbl[])
        n446 = Unbundle By Name(w1155) -> ("Table"=w1170:string[][], "daemon reference"=w1176:refnum<k5>, "Config"=w1168:string[][])
        n447 = call "Select_Table_Vaule Enable_Disable.vi"("Action"=w1171, "Table"=w1170) -> ("Enable"=w1169:bool)  [unwired: 8 in, 1 out]
        n448 = case shown="假" w1169 {
          tunnel: w1176 -> [w1184 w1206]
          tunnel: [w1184 w1206] -> w1154
          tunnel: [w1183 w1197] -> w1172
          tunnel: w1171 -> [_ w1204]
          tunnel: w1170 -> [_ w1207]
          tunnel: w1168 -> [_ _]
          tunnel: [_ w1196] -> w1160
          tunnel: w1158 -> [_ w1195]
          tunnel: w1157 -> [_ w1194]
          tunnel: [_ w1190] -> w1156
          tunnel: [w1182 w1186] -> w1134
          tunnel: [w1182 w1185] -> w1135
          frame False {
            w1183 = "Skip" ("software string")
            n449 = Initialize Array(w1183, 3 ("维数大小")) -> (w1182:string[])
          }
          frame True {
            w1198 = string[] ["Initialisation_DDM_Pressure_corrected", "Initialisation_DDM_Real_Power", "Initialisation_Delta_V"]
            n450 = call "AW_Calculate_Tester_Parameter_Initialisation.vi"("Tester Parameter"=w1194, "DDM Parameter"=w1195) -> ("Calculate Tester Parameter"=w1196:dbl[])  [unwired: 9 in]
            n451 = Number To Fractional String(number=w1196) -> (F-format string=w1185:string[])  [unwired: 3 in]
            n452 = Interleave 1D Arrays(w1198, w1185) -> (w1201:string[])
            n453 = Array To Spreadsheet String(delimiter (Tab)=";" ("分隔符(Tab)"), array=w1201, 3:"" ("格式字符串")) -> (spreadsheet string=w1197:string)
            n454 = Build Array (concatenate)(w1204, w1198) -> (w1205:string[])
            n455 = Build Array (concatenate)("", w1185) -> (w1203:string[])
            n456 = for {
              tunnel: w1207 -> [w1213]
              tunnel: w1203 -> [w1211] mode=indexing
              tunnel: w1205 -> [w1210] mode=indexing
              tunnel: [w1209] -> w1193 mode=indexing
              tunnel: [w1208] -> w1187 mode=indexing
              w1218 = "UIdisplay" ("Process (\"\" - local)")
              n457 = call "Select_Table_Vaule.vi"("Vaule"=w1211, "Action"=w1210, "Table"=w1213) -> ("Result"=w1209:bool, "vaule"=w1212:string[])  [unwired: 7 in]
              n458 = Append True/False String(1:w1209, 2:"FAIL" ("真字符串"), 3:"PASS" ("真字符串")) -> (0:w1208:string)  [unwired: 1 in]
              n459 = Build Array (concatenate)(w1212, w1211, w1208) -> (w1217:string[])
              n460 = Flatten To XML(anything=w1217) -> (xml string=w1216:string)
              n461 = call "AMC Send Local Message.vi"("Process (\"\" - local)"=w1218, "Message Value"=w1216, "Message Name"=w1218) -> ()  [unwired: 7 in, 2 out]
            }
            n462 = Delete From Array(array=w1193, length=1 ("长度"), index=0 ("索引")) -> (array with subset deleted=w1190:bool[])  [unwired: 1 out]
            n463 = Delete From Array(array=w1187, length=1 ("长度"), index=0 ("索引")) -> (array with subset deleted=w1186:string[])  [unwired: 1 out]
          }
        }
        n464 = Unbundle By Name(w1144) -> ("MES bool"=w1148:refnum<vi>)
        n465 = call "HD_Config.vi"("Step"=enum16{"Initial", "Write", "Read"}."Read") -> ("HD Config out"=w1147:T11)  [unwired: 9 in, 1 out]
        n466 = Unbundle By Name(w1147) -> ("Fail_resume_mode"=w1149:bool)
        n467 = property class="Bool (严格)"(reference=w1148) -> ("Value"=w1150:bool)  [unwired: 1 in, 2 out]
        n468 = call <vilib>:"Space Constant.vi"() -> ("String"=w1174:string)
        n469 = Not(x=w1150) -> (.not. x?=w1151:bool)
        n470 = Concatenate Strings(w1171, w1174, w1172) -> (w1173:string)
        n471 = Or(x=w1149, y=w1151) -> (x .or. y?=w1152:bool)
        n472 = Unbundle By Name(w1159) -> ("Initialisation.DDM_Parameter_status"=w1167:bool[], "Initialisation.Get_Tester_Parameter_status"=w1166:bool[])
        n473 = Index Array(array=w1135) -> (element #1=w1141:string, element #2=w1140:string, element #3=w1139:string)  [unwired: 3 in]
        n474 = Index Array(array=w1134) -> (element #1=w1136:string, element #2=w1137:string, element #3=w1138:string)  [unwired: 3 in]
        n475 = Bundle By Name(cluster=w1155, "daemon reference"=w1154, "Initialisation.Calculated Parameter - DDM Pressure Corrected"=w1141, "Initialisation.Calculated Parameter - DDM Real Power"=w1140, "Initialisation.Calculated Parameter - Delta V"=w1139, "Initialisation_Status.Calculated Parameter - DDM Pressure Corrected"=w1136, "Initialisation_Status.Calculated Parameter - DDM Real Power"=w1137, "Initialisation_Status.Calculated Parameter - Delta V"=w1138) -> (w1153:T1)
        n476 = Build Array (concatenate)(w1167, w1166, w1156) -> (w1165:bool[])
        n477 = Bundle By Name(cluster=w1159, "Initialisation.Cal_Tester_Parameter"=w1160, "Initialisation.Cal_Tester_Parameter_status"=w1156) -> (w1175:T3)
        n478 = And Array Elements(Boolean array=w1165) -> (logical AND=w1142:bool)
        n479 = Select(t=TRUE, s=w1152, f=w1142) -> (s? t:f=w1143:bool)
        n480 = call "LogStatus.vi"("error in (no error)"=w1179, "last message"=w1177, "message"=w1173) -> ("error  out"=w1178:errorcluster)  [unwired: 8 in]
        n481 = Select(t="Calibration_BEMF", s=w1143, f="Finalization_NG_unit") -> (s? t:f=w1161:string)
      }
      frame "Reflashing" {
        w1234 = "UIdisplay" ("Process (\"\" - local)")
        n482 = Unbundle By Name(w1219) -> ("Table"=w1233:string[][])
        n483 = call "Select_Table_Vaule Enable_Disable.vi"("Action"=w1231, "Table"=w1233) -> ("Enable"=w1225:bool)  [unwired: 8 in, 1 out]
        n484 = case shown="真" w1225 {
          tunnel: w1248 -> [w1251 w1264]
          tunnel: w1247 -> [_ w1263]
          tunnel: w1231 -> [w1250 w1262]
          tunnel: [w1251 w1260] -> w1246
          tunnel: w1245 -> [w1253 w1259]
          tunnel: [w1253 w1258] -> w1244
          tunnel: [w1252 w1256] -> w1243
          tunnel: [w1250 w1257] -> w1228
          tunnel: w1232 -> [w1252 w1256]
          tunnel: [w1249 w1254] -> w1220
          tunnel: w1219 -> [w1249 w1255]
          frame False {
          }
          frame True {
            n485 = call "LogStatus.vi"("error in (no error)"=w1264, "last message"=w1263, "message"=w1262) -> ("error  out"=w1261:errorcluster)  [unwired: 8 in]
            n486 = call "1.0.2_UUT_Reflashing.vi"("error in (no error)"=w1261, "Data in"=w1255, "Message Queue out"=w1259) -> ("error out"=w1260:errorcluster, "Flow"=w1257:string, "Data out"=w1254:T1, "Message Queue Out"=w1258:T4)  [unwired: 5 in]
          }
        }
        n487 = Select(t="Enable" ("元素"), s=w1225, f="Disable" ("元素")) -> (s? t:f=w1222:string)
        n488 = Flush Queue(queue=w1244) -> (queue out=w1221:T4)  [unwired: 1 in, 2 out]
        n489 = call "Select_Table_Vaule.vi"("Vaule"=w1222, "Action"=w1231, "Table"=w1233) -> ("Result"=w1241:bool, "vaule"=w1240:string[])  [unwired: 7 in]
        n490 = Append True/False String(1:w1241, 2:"FAIL" ("真字符串"), 3:"PASS" ("真字符串")) -> (0:w1239:string)  [unwired: 1 in]
        n491 = Build Array (concatenate)(w1240, w1222, w1239) -> (w1237:string[])
        n492 = Flatten To XML(anything=w1237) -> (xml string=w1238:string)
        n493 = call "AMC Send Local Message.vi"("Process (\"\" - local)"=w1234, "Message Value"=w1238, "Message Name"=w1234) -> ()  [unwired: 7 in, 2 out]
        n494 = Equal?(x=w1228, y="Disconnect_UUT") -> (x = y?=w1230:bool)
        n495 = Equal?(x=w1228, y="Error" ("Message Name")) -> (x = y?=w1226:bool)
        n496 = Or(x=w1230, y=w1226) -> (x .or. y?=w1227:bool)
      }
    }
    n497 = call "Stop.vi"("Step"=enum16{"Initial", "Write", "Read"}."Read") -> ("Stop Out"=w30:bool)  [unwired: 9 in, 1 out]
    n498 = call "Exit.vi"("Step"=enum16{"Initial", "Write", "Read"}."Read" ("step")) -> ("Exit Out"=w29:bool)  [unwired: 9 in, 1 out]
    n499 = call "6-AlarmStatus.vi"("Step"=enum16{"Initial", "Write", "Read"}."Read") -> ("AlarmValue Out"=w24:bool[])  [unwired: 9 in, 1 out]
    n500 = Or Array Elements(Boolean array=w24) -> (logical OR=w23:bool)
    n501 = call "AMC Run Step.vi"("Message Queue In"=w49, "Message Name"=w38, "Message Value"=w36, "error in (no error)"=w44, "Mli/Sig"=FALSE) -> ("Message Queue Out"=w48:T4, "error out"=w43:errorcluster)  [unwired: 13 in]
    n502 = Compound Arithmetic op=OR(w32, w30, w29, w23) -> (w31:bool)
  }
  "Message Queue Out" <- w12
  "error out" <- w11
  "Data" <- w15
  "Flow" <- w14
  "Data out" <- w8
